vi "_calc_IFoutput.vi"(11 "Calc_IFout":T1={"Th"=299.0, "Tc"=83.0, "BW (MHz)"=40.0, "NS_output_data"=path "L:/cartridge/assembly/SN03/03-13/110628_WCADSB_P0/YIG_938.00_120_110628_WCADSB_P0aNS.csv", "Rx_output_data"=path "L:/cartridge/assembly/SN03/03-13/110628_WCADSB_P0/YIG_802.00_120_110628_WCADSB_P0m.csv", "NS_ENR"=path "Z:/Labview_ALMA/MIX10/110627_IFBOX/NS_ENR_44421726.csv", "SAVE"=TRUE, "IFB_NS_AMP(filename)"="", "IFB_INPUT_CBL(filename) "=""}) -> (1 "出力文字列":string, 3 "Calc_IFout 2":T1={"Th"=299.0, "Tc"=83.0, "BW (MHz)"=40.0, "NS_output_data"=path "L:/cartridge/assembly/SN03/03-13/110628_WCADSB_P0/YIG_938.00_120_110628_WCADSB_P0aNS.csv", "Rx_output_data"=path "L:/cartridge/assembly/SN03/03-13/110628_WCADSB_P0/YIG_802.00_120_110628_WCADSB_P0m.csv", "NS_ENR"=path "Z:/Labview_ALMA/MIX10/110627_IFBOX/NS_ENR_44421726.csv", "SAVE"=TRUE, "IFB_NS_AMP(filename)"="", "IFB_INPUT_CBL(filename) "=""})   [LabVIEW 2017]
uses:
  <vilib>/Utility/file.llb/Read From Spreadsheet File (DBL).vi
  <vilib>/Utility/file.llb/Read From Spreadsheet File (string).vi
  Instance           2 22Saved   _calc_IFoutput .vi
  Instance           3 22Saved   _calc_IFoutput .vi
  Instance           4 22Saved   _calc_IFoutput .vi
  Instance           5 22Saved   _calc_IFoutput .vi
  Instance           6 22Saved   _calc_IFoutput .vi
  <vilib>/express/express shared/transition.llb/Dynamic To Waveform Array.vi
  <vilib>/express/express arith-compare/Formula/Block/exnFormulaBlock how many pts in the wave.vi
  <vilib>/express/express shared/ex_Modify Signal Name.vi
  <vilib>/express/express shared/transition.llb/Waveform Array To Dynamic.vi
  Instance          14 22Saved   _calc_IFoutput .vi
  Instance          13 22Saved   _calc_IFoutput .vi
  Instance           8 22Saved   _calc_IFoutput .vi
  Instance          27 22Saved   _calc_IFoutput .vi
  Instance          25 22Saved   _calc_IFoutput .vi
  Instance          24 22Saved   _calc_IFoutput .vi
  Instance          23 22Saved   _calc_IFoutput .vi
  Instance           9 22Saved   _calc_IFoutput .vi
  <vilib>/express/express arith-compare/Formula/XNode/ExpressFormulaBlockNode.xnode
  <vilib>/gmath/NI_Gmath.lvlib
panel:
  out "配列 2":dbl[][](array[numeric])=[[3.8, -17.12272, -18.81083, -15.55195, -27.42913, -0.8529618823529413, 2646.4699989426, 27.159200000349998, 21.830696906606043], [3.85, -17.57263, -19.57423, -15.61331, -27.39271, -0.8547822352941177, 2630.0700003280003, 27.222799998728, 21.827656711269793], [3.9, -17.18393, -19.46044, -15.25915, -26.95194, -0.8662073529411765, 2669.6499992084, 27.104500002366002, 21.82485128829734], [3.95, -16.20817, -18.50417, -14.57025, -26.2268, -0.8667218823529415, 2730.9599987738, 27.08000000049, 21.822294447827726], [4.0, -15.03429, -17.26599, -13.90883, -25.64848, -0.882467, 2669.1500012362003, 27.084199999916, 21.82], [4.05, -14.82404, -17.0148, -13.89065, -25.63071, -0.881857, 2537.9100026248, 27.120499999274, 21.817975444814163], [4.1, -14.67198, -16.88321, -13.75199, -25.74328, -0.8925589411764706, 2521.6700003248, 26.984300002724, 21.81620304171403], [4.15, -13.82526, -16.05723, -13.35155, -25.22083, -0.8985360624999998, 2529.2999998474, 26.948000000726, 21.81465874000436], [4.2, -13.29308, -15.43659, -13.22012, -25.15282, -0.901060705882353, 2508.1700004226, 26.933300000294, 21.81331848898993], [4.25, -13.22027, -15.33436, -13.24037, -25.05297, -0.9175218823529412, 2527.4499996144, 26.893400000798, 21.812158237975495], [4.3, -13.31871, -15.44813, -13.02047, -24.85233, -0.9171115294117648, 2617.4499981999998, 26.800200001864, 21.81115393626583], [4.35, -13.69981, -15.96198, -12.64103, -24.38364, -0.9331128235294116, 2655.3199992426003, 26.946899997065998, 21.810281533165693], [4.4, -13.88617, -16.39624, -12.56773, -24.29817, -0.9225989999999998, 2612.6100008542003, 26.89840000097, 21.809516977979857], [4.45, -14.02675, -16.71935, -12.80309, -24.58885, -0.9326420000000001, 2578.7800006766, 26.85540000086, 21.808836220013085], [4.5, -14.20917, -16.89711, -12.97901, -24.88372, -0.9390088823529412, 2494.6900016818004, 26.752700002054002, 21.808215208570147], [4.55, -14.08214, -16.69081, -12.94844, -24.93315, -0.948472375, 2435.9600011746, 26.64920000207, 21.807629892955802], [4.6, -14.17748, -16.75517, -13.06879, -25.00575, -0.9494775294117647, 2433.2400000544, 26.427400004436, 21.80705622247482], [4.65, -14.20809, -16.81901, -13.13087, -25.16717, -0.9524575882352941, 2443.0399998039998, 26.363500001278, 21.80647014643197], [4.7, -13.73884, -16.38887, -13.13099, -25.03512, -0.9655740588235294, 2433.8500001838, 26.45199999823, 21.805847614132016], [4.75, -13.52419, -16.15298, -13.15192, -24.9704, -0.9653059411764703, 2516.0199983566, 26.454299999954, 21.805164574879722], [4.8, -13.5663, -16.20232, -13.10517, -24.80095, -0.976770176470588, 2562.8099990642, 26.343600002214, 21.804396977979856], [4.85, -13.97629, -16.65383, -13.30715, -25.25404, -0.9746549411764707, 2478.4000016882, 26.311400000644, 21.803520772737187], [4.9, -14.61364, -17.38417, -13.78671, -25.66877, -0.988881117647059, 2394.9800016684003, 26.140100003426, 21.802511908456477], [4.95, -14.4268, -17.25931, -13.81209, -25.80221, -0.9904888125, 2426.7199993652, 26.145399999894, 21.801346334442492], [5.0, -13.84685, -16.67325, -13.20797, -25.09457, -0.9986477647058825, 2402.3700004869997, 26.405599994796, 21.8], [5.05, -14.28601, -17.05717, -13.45101, -25.54052, -1.004, 2304.7500019524, 26.325300001606, 21.798457844989954], [5.1, -14.91876, -17.64101, -13.96415, -26.02207, -1.0068823529411761, 2324.9199995966, 26.481899996868, 21.796740771498058], [5.15, -15.14906, -17.85047, -14.16308, -26.17572, -1.0180588235294117, 2408.1599983352, 26.271100004216002, 21.794878672166195], [5.2, -14.66069, -17.39484, -13.82115, -25.80543, -1.0208823529411764, 2393.2200002987997, 26.329699998827998, 21.792901439636257], [5.25, -13.73691, -16.45963, -13.31747, -25.36704, -1.028, 2326.370001337, 26.25120000157, 21.790838966550133], [5.3, -13.70664, -16.41934, -13.34713, -25.41262, -1.0291176470588232, 2366.9299991887997, 26.28519999932, 21.78872114554971], [5.35, -14.26567, -16.97919, -13.7311, -25.69348, -1.042, 2383.6799996649997, 26.357999998544, 21.78657786927688], [5.4, -14.42577, -17.17993, -13.89956, -26.00954, -1.046, 2311.580001442, 26.332800000503997, 21.784439030373523], [5.45, -14.3035, -17.10186, -13.87839, -26.01249, -1.0538235294117648, 2274.08000075, 26.241800001820003, 21.782334521481534], [5.5, -14.13436, -16.92141, -13.94402, -26.09274, -1.0542500000000001, 2305.5199993712, 26.224000000356, 21.780294235242803], [5.55, -14.09064, -16.88934, -13.93655, -25.97309, -1.0640588235294117, 2314.2099998262, 26.143600001608, 21.778348064299216], [5.6, -14.13487, -16.88146, -13.83602, -26.02727, -1.0725882352941176, 2258.5000011142, 26.194499998982, 21.776525901292658], [5.65, -14.0179, -16.75543, -13.67357, -25.85477, -1.0641764705882353, 2249.6300001774002, 26.303699997816, 21.774857638865026], [5.7, -13.742, -16.4761, -13.49645, -25.65245, -1.085294117647059, 2312.4099987443997, 26.495899996156, 21.7733731696582], [5.75, -13.63401, -16.37811, -13.62051, -25.66763, -1.0879411764705882, 2296.9000003102, 26.546799998982, 21.77210238631407], [5.8, -13.9966, -16.7347, -14.08119, -26.28417, -1.0975294117647059, 2229.90000134, 26.494200001052, 21.77107518147453], [5.85, -14.3776, -17.12208, -14.29554, -26.5205, -1.0957647058823532, 2219.9900001981996, 26.459700000690002, 21.770321447781463], [5.9, -14.33998, -17.0836, -14.21864, -26.41191, -1.0961250000000002, 2230.8999997818, 26.353800002118, 21.76987107787676], [5.95, -14.05573, -16.80771, -13.83659, -26.01129, -1.106764705882353, 2262.3899993702, 26.544199996192, 21.76975396440231], [6.0, -14.15222, -16.88773, -14.02318, -26.27665, -1.110529411764706, 2218.8600008706003, 26.523000000424, 21.77], [6.05, -14.42877, -17.16834, -14.46916, -26.71696, -1.1207647058823527, 2201.7700003418, 26.482100000818, 21.770629425226016], [6.1, -14.82458, -17.54857, -14.74361, -26.94142, -1.1145882352941179, 2213.8099997592, 26.528199999077998, 21.77162387229374], [6.15, -14.43141, -17.15023, -14.50576, -26.74506, -1.1284117647058822, 2219.209999892, 26.454400001476, 21.77295532133086], [6.2, -13.88065, -16.61938, -14.37111, -26.68039, -1.128235294117647, 2179.0500008032004, 26.372000001648, 21.77459575246504], [6.25, -13.64365, -16.3979, -14.22502, -26.5427, -1.135764705882353, 2168.7100002068, 26.34000000064, 21.77651714582397], [6.3, -13.8741, -16.64741, -14.49609, -26.71762, -1.14025, 2200.3899993664, 26.582799995143997, 21.77869148153533], [6.35, -14.26957, -17.0322, -14.86186, -27.19956, -1.1440588235294114, 2204.6199999154, 26.591799999819997, 21.781090739726796], [6.4, -15.05829, -17.80809, -15.42064, -27.71206, -1.1539411764705882, 2184.0000004124, 26.470100002434, 21.78368690052605], [6.45, -14.96881, -17.71266, -15.38201, -27.65482, -1.1564705882352941, 2195.249999775, 26.481999999762, 21.786451944060772], [6.5, -14.62204, -17.38934, -15.02896, -27.20097, -1.1578823529411766, 2242.3699990575997, 26.306800003503998, 21.789357850458643], [6.55, -14.93231, -17.69407, -15.10335, -27.40647, -1.164235294117647, 2205.1300007448003, 26.310299999930002, 21.79237659984734], [6.6, -15.6833, -18.43714, -15.87043, -28.20904, -1.172, 2152.5300010520004, 26.339899999408, 21.795480172354544], [6.65, -16.11679, -18.87216, -16.20987, -28.58401, -1.1799411764705883, 2167.9899996908, 26.356799999661998, 21.798640548107933], [6.7, -15.71971, -18.45462, -15.76916, -28.0619, -1.185, 2201.939999321, 26.396499999206, 21.80182970723519], [6.75, -15.0464, -17.78941, -15.52487, -27.82688, -1.195, 2182.7000003847998, 26.399599999938, 21.805019629863992], [6.8, -15.48116, -18.24106, -16.05464, -28.38039, -1.2004117647058823, 2165.3400003472, 26.28360000232, 21.808182296122023], [6.85, -16.22272, -18.99162, -16.63654, -28.97924, -1.201, 2225.439998798, 26.274900000174, 21.81128968613696], [6.9, -15.67766, -18.42345, -16.38983, -28.69264, -1.2098823529411764, 2234.0299998282003, 26.270200000094, 21.814313780036482], [6.95, -15.36656, -18.07411, -15.9862, -28.27599, -1.2114117647058824, 2165.6200013682, 26.381899997766002, 21.817226557948267], [7.0, -15.74528, -18.46492, -16.29495, -28.63586, -1.218, 2163.1900000486003, 26.272700002184, 21.82], [7.05, -16.00173, -18.75385, -16.78861, -29.11719, -1.2230588235294118, 2187.8999995058, 26.169500002063998, 21.82260695410598], [7.1, -15.95475, -18.70909, -16.46813, -28.80718, -1.2295882352941179, 2186.0500000370002, 26.233599998718, 21.825023739326973], [7.15, -15.74736, -18.51188, -16.0888, -28.41011, -1.228, 2172.6600002677997, 26.140200001868, 21.827227542510375], [7.2, -15.79896, -18.55205, -16.49574, -28.80938, -1.2389411764705882, 2190.1299996506, 26.035800002088, 21.82919555050358], [7.25, -16.55221, -19.29029, -17.09613, -29.38037, -1.2441250000000001, 2230.579999191, 25.944300001829998, 21.830904950153982], [7.3, -16.63515, -19.36656, -17.1755, -29.45088, -1.2501764705882352, 2201.3800005840003, 26.127399996338003, 21.83233292830897], [7.35, -16.28817, -19.02285, -17.12399, -29.45578, -1.2507058823529413, 2186.5600002964, 26.014300002261997, 21.833456671815934], [7.4, -15.91257, -18.66145, -16.74209, -29.02037, -1.2591176470588235, 2205.0399996304, 26.029399999698, 21.834253367522273], [7.45, -15.41844, -18.14403, -16.48895, -28.79334, -1.2650588235294118, 2206.9099999626, 25.964200001304, 21.83470020227537], [7.5, -15.41264, -18.10839, -16.57757, -28.91563, -1.273764705882353, 2195.2200002338, 26.019099998902, 21.834774362922627], [7.55, -15.98175, -18.66501, -16.9447, -29.22746, -1.2748235294117647, 2200.019999904, 25.824000003902, 21.834453036311427], [7.6, -15.94066, -18.66749, -17.16323, -29.42903, -1.2809411764705882, 2244.7899991045997, 25.813600000208, 21.833713409289167], [7.65, -15.86338, -18.63036, -17.30867, -29.55716, -1.2772500000000002, 2247.2699999504, 25.856499999142, 21.83253266870324], [7.7, -15.93995, -18.73317, -17.33017, -29.58961, -1.2859411764705884, 2238.1100001832, 25.730900002511998, 21.83088800140104], [7.75, -15.60121, -18.40257, -17.32444, -29.63481, -1.299588235294118, 2218.8700003848, 25.69040000081, 21.828756594229954], [7.8, -15.52939, -18.3085, -17.34604, -29.61109, -1.2968235294117643, 2243.669999504, 25.680500000198, 21.82611563403738], [7.85, -15.91931, -18.69063, -17.7087, -29.96924, -1.3002352941176467, 2245.9399999546, 25.647100000667997, 21.8229423076707], [7.9, -16.06734, -18.84154, -18.21152, -30.51118, -1.3056250000000003, 2218.990000539, 25.507500002792, 21.819213801977316], [7.95, -16.2394, -19.01631, -18.39538, -30.77489, -1.313764705882353, 2222.539999929, 25.53849999938, 21.81490730380462], [8.0, -16.0832, -18.82693, -18.18621, -30.42877, -1.3231176470588235, 2253.7699993754, 25.421100002348, 21.81], [8.05, -15.9397, -18.65948, -18.21682, -30.46989, -1.332941176470588, 2276.81, 25.2307, 21.804486508350074], [8.1, -16.44804, -19.16853, -18.58308, -30.82861, -1.335, 2261.15, 25.2839, 21.79843117039837], [8.15, -16.97081, -19.72537, -19.0693, -31.4089, -1.3383529411764703, 2262.78, 25.2973, 21.79191575862764], [8.2, -16.87192, -19.67071, -19.41342, -31.67662, -1.348647058823529, 2301.63, 25.0593, 21.78502204552063], [8.25, -17.21139, -20.03537, -19.67853, -31.95149, -1.3514117647058825, 2289.19, 24.9943, 21.777831803560098], [8.3, -17.29203, -20.11014, -19.70503, -32.02495, -1.352470588235294, 2259.82, 25.224, 21.77042680522879], [8.35, -16.73358, -19.52565, -19.51154, -31.79005, -1.357705882352941, 2266.94, 24.9458, 21.76288882300946], [8.4, -16.47973, -19.26356, -19.55496, -31.8567, -1.365235294117647, 2296.06, 24.8175, 21.75529962938486], [8.45, -16.96765, -19.74245, -20.13428, -32.43519, -1.3692499999999999, 2317.78, 24.8136, 21.747740996837745], [8.5, -17.89289, -20.67773, -21.16278, -33.47596, -1.377, 2296.65, 24.8236, 21.740294697850857], [8.55, -18.31942, -21.11132, -21.53435, -33.99178, -1.377882352941177, 2303.42, 24.7167, 21.73304250490695], [8.6, -17.91342, -20.68657, -21.06001, -33.3284, -1.3864117647058825, 2312.28, 24.5475, 21.72606619048878], [8.65, -17.50286, -20.31712, -20.86753, -33.1991, -1.3915882352941176, 2326.39, 24.57, 21.719447527079094], [8.7, -17.7744, -20.60603, -21.46811, -33.89479, -1.3978823529411766, 2298.81, 24.1647, 21.713268287160645], [8.75, -17.86462, -20.69869, -21.66053, -34.15056, -1.4036470588235284, 2302.5, 24.3807, 21.707610243216184], [8.8, -17.71743, -20.57318, -21.35601, -33.74465, -1.4073529411764707, 2313.14, 24.5441, 21.702555167728462], [8.85, -17.94226, -20.78062, -21.59592, -34.02443, -1.4161875, 2345.93, 24.4626, 21.698184833180232], [8.9, -18.34472, -21.16955, -22.16719, -34.56456, -1.4160588235294116, 2339.53, 24.3008, 21.694581012054247], [8.95, -18.04812, -20.86419, -21.99622, -34.46492, -1.4309411764705886, 2338.73, 24.441, 21.69182547683325], [9.0, -17.40652, -20.21983, -21.48231, -33.78672, -1.4215882352941176, 2358.4, 24.3139, 21.69], [9.05, -17.24231, -20.07737, -21.48494, -33.82899, -1.4349411764705877, 2366.74, 24.1072, 21.689155762493723], [9.1, -17.74864, -20.56868, -21.94918, -34.39316, -1.4335882352941178, 2338.76, 24.3848, 21.689221579079543], [9.15, -18.4194, -21.25906, -22.30343, -34.74111, -1.453, 2315.94, 24.6737, 21.690095672979066], [9.2, -18.22584, -21.06735, -22.19776, -34.35875, -1.451705882352941, 2343.85, 24.5305, 21.69167626741389], [9.25, -17.60283, -20.47247, -21.72121, -33.8754, -1.4561250000000001, 2374.94, 24.293, 21.69386158560562], [9.3, -17.285, -20.1526, -21.26908, -33.42764, -1.4694117647058822, 2365.34, 24.4681, 21.69654985077586], [9.35, -17.46603, -20.32564, -21.38399, -33.71154, -1.4681764705882352, 2354.91, 24.3401, 21.699639286146212], [9.4, -17.69275, -20.52774, -21.7712, -34.03559, -1.4925882352941173, 2368.34, 24.4059, 21.703028114938277], [9.45, -17.89483, -20.70066, -21.80327, -33.93689, -1.473, 2362.78, 24.6405, 21.706614560373655], [9.5, -17.75022, -20.53087, -21.69907, -34.00557, -1.507411764705883, 2338.42, 24.6167, 21.710296845673955], [9.55, -17.66432, -20.45212, -21.90227, -34.10663, -1.4951764705882342, 2333.22, 24.5527, 21.713973194060774], [9.6, -17.65736, -20.44671, -21.78109, -33.9852, -1.522470588235294, 2332.23, 24.4424, 21.717541828755717], [9.65, -17.73314, -20.5128, -21.7289, -33.99685, -1.517823529411764, 2328.62, 24.6084, 21.720900972980388], [9.7, -17.4669, -20.25952, -21.67133, -33.91276, -1.525588235294116, 2351.26, 24.2804, 21.723948849956383], [9.75, -17.76851, -20.58019, -22.0069, -34.18419, -1.5647058823529412, 2359.86, 24.4864, 21.72658368290531], [9.8, -18.45745, -21.3164, -22.66344, -34.81685, -1.5282499999999999, 2394.51, 24.4116, 21.72870369504877], [9.85, -18.74849, -21.60512, -23.1135, -35.51059, -1.5908235294117645, 2378.32, 24.3508, 21.73020710960837], [9.9, -18.03912, -20.85912, -22.19721, -34.52363, -1.5453529411764708, 2394.59, 24.2431, 21.730992149805704], [9.95, -17.9064, -20.68631, -21.64287, -33.76706, -1.6109999999999993, 2382.76, 24.4119, 21.730957038862382], [10.0, -18.76585, -21.52492, -22.34931, -34.56586, -1.5900588235294104, 2349.48, 24.4835, 21.73], [10.05, -19.5962, -22.32853, -22.9941, -35.31366, -1.6072352941176506, 2367.23, 24.3783, 21.72805419167504], [10.1, -19.6706, -22.4559, -22.82671, -35.05968, -1.6390588235294121, 2371.78, 24.5145, 21.72519251328346], [10.15, -19.60253, -22.38713, -22.75759, -35.06578, -1.594882352941177, 2400.96, 24.3435, 21.721522799456107], [10.2, -19.78752, -22.57098, -23.06087, -35.44369, -1.681875, 2420.45, 24.0411, 21.71715288482381], [10.25, -20.0526, -22.84692, -23.63574, -35.82155, -1.6011764705882354, 2439.32, 23.8385, 21.712190604017422], [10.3, -19.54974, -22.37162, -23.29077, -35.54749, -1.6889411764705888, 2425.46, 24.0043, 21.70674379166777], [10.35, -19.60772, -22.45374, -23.18082, -35.44497, -1.6339411764705871, 2402.21, 24.136, 21.700920282405693], [10.4, -19.77289, -22.58667, -23.44011, -35.6872, -1.6639411764705916, 2403.53, 24.1481, 21.69482791086204], [10.45, -19.79049, -22.58858, -23.37076, -35.6931, -1.6936470588235286, 2410.86, 24.2845, 21.688574511667635], [10.5, -19.04526, -21.81113, -22.73856, -34.75031, -1.6280000000000006, 2432.24, 24.1535, 21.68226791945333], [10.55, -18.56993, -21.3308, -22.71269, -34.42597, -1.7282941176470574, 2457.87, 23.9651, 21.676015968849956], [10.6, -18.81393, -21.59022, -23.3418, -35.09374, -1.627000000000001, 2472.89, 23.7868, 21.669926494488355], [10.65, -19.22983, -22.00177, -23.51241, -35.50699, -1.7109411764705882, 2463.24, 23.8037, 21.664107330999364], [10.7, -19.31875, -22.05797, -23.32962, -35.59218, -1.6540588235294145, 2430.32, 23.8234, 21.658666313013825], [10.75, -19.05511, -21.80451, -23.11849, -35.37068, -1.6625882352941161, 2456.31, 23.8229, 21.653711275162575], [10.8, -19.3566, -22.10467, -23.36395, -35.42174, -1.644, 2526.85, 23.8448, 21.64935005207645], [10.85, -19.0206, -21.80983, -23.26736, -35.08837, -1.653941176470586, 2539.44, 23.6902, 21.645690478386292], [10.9, -18.31242, -21.08287, -22.35121, -34.319, -1.678058823529411, 2516.98, 23.7731, 21.642840388722938], [10.95, -18.58308, -21.32811, -22.20398, -34.26554, -1.6376470588235292, 2511.94, 23.7372, 21.64090761771723], [11.0, -19.33065, -22.06466, -22.81771, -34.93946, -1.6834705882352938, 2495.74, 23.8567, 21.64], [11.05, -19.70611, -22.43568, -23.07443, -35.23765, -1.6487058823529408, 2471.76, 23.7069, 21.64017747080613], [11.1, -19.03199, -21.75445, -22.37182, -34.36297, -1.6840588235294118, 2484.68, 23.978, 21.64130836778662], [11.15, -18.20851, -20.94228, -21.81273, -33.92755, -1.65975, 2530.13, 23.6561, 21.643213129196518], [11.2, -18.60047, -21.36138, -22.13935, -34.33841, -1.7035294117647042, 2549.97, 23.6568, 21.645712193290862], [11.25, -19.51813, -22.27067, -22.85502, -34.9773, -1.6814705882352947, 2588.62, 23.5463, 21.6486259983247], [11.3, -20.00388, -22.73884, -23.1136, -35.31568, -1.7118823529411817, 2547.84, 23.759, 21.651774982553068], [11.35, -20.09303, -22.81332, -23.00719, -35.05995, -1.7251176470588228, 2534.41, 23.8176, 21.654979584231015], [11.4, -19.73824, -22.45692, -22.58862, -34.67323, -1.7182352941176506, 2543.99, 23.8915, 21.658060241613576], [11.45, -19.50205, -22.22064, -22.28212, -34.3972, -1.75829411764706, 2558.35, 23.9421, 21.660837392955802], [11.5, -19.44096, -22.15222, -22.1292, -34.22024, -1.7096470588235253, 2566.32, 23.8669, 21.663131476512728], [11.55, -19.53986, -22.21978, -22.16747, -34.08258, -1.805937499999999, 2585.21, 23.691, 21.664762930539403], [11.6, -19.66825, -22.31744, -22.50284, -34.28826, -1.7306470588235299, 2620.79, 23.6435, 21.665552193290864], [11.65, -20.25282, -22.89179, -22.68607, -34.6127, -1.833705882352942, 2632.79, 23.8005, 21.665319703022153], [11.7, -20.71909, -23.33487, -22.77796, -34.75574, -1.7838235294117686, 2608.38, 23.9055, 21.663885897988315], [11.75, -20.60419, -23.22526, -22.42747, -34.3851, -1.7971764705882394, 2594.61, 24.0102, 21.661071216444395], [11.8, -19.96298, -22.55664, -21.58718, -33.45363, -1.8430588235294112, 2639.94, 23.9067, 21.656696096645433], [11.85, -19.76787, -22.40006, -21.42269, -33.29006, -1.7760588235294126, 2643.51, 23.9414, 21.650580976846467], [11.9, -20.8505, -23.49592, -22.22725, -34.22635, -1.8767647058823524, 2626.67, 23.9677, 21.642546295302548], [11.95, -21.60192, -24.17152, -22.54207, -34.5773, -1.7737499999999975, 2639.97, 23.9508, 21.63241249026871], [12.0, -21.64507, -24.22899, -22.299, -34.30385, -1.8910588235294117, 2735.39, 23.7742, 21.62], [12.05, -21.23121, -23.79945, -21.79121, -33.84, -1.7987058823529407, 2735.72, 24.015, 21.60517967510045], [12.1, -20.95311, -23.50938, -21.58213, -33.39882, -1.879823529411763, 2675.38, 24.0166, 21.588024015570067], [12.15, -20.98547, -23.59292, -21.93953, -33.86782, -1.885, 2668.38, 24.2213, 21.56865593375783], [12.2, -20.95372, -23.58369, -22.31312, -34.16981, -1.8179411764705862, 2763.59, 23.8837, 21.54719834201274]]
  in  "タブ制御器":enum32{"YIGファイル", "配列"}(tab)
  out "Trx(K)":dbl=258.9214466673217 format="%#_5g"
  out "PrxCold(dBm)":dbl=-6.962263655715082 format="%#_4g"
  out "PrxHOT(dBm)":dbl=-4.835796517513394 format="%#_4g"
  out "XYグラフ 4":cluster{"データ配列":dbl[], "データ配列":dbl[]}[](graph)=[{"データ配列"=[4.0, 4.1, 4.2, 4.3, 4.4, 4.5, 4.6, 4.7, 4.8, 4.9, 5.0, 5.1, 5.2, 5.3, 5.4, 5.5, 5.6, 5.7, 5.8, 5.9, 6.0, 6.1, 6.2, 6.3, 6.4, 6.5, 6.6, 6.7, 6.8, 6.9, 7.0, 7.1, 7.2, 7.3, 7.4, 7.5, 7.6, 7.7, 7.8, 7.9, 8.0, 8.1, 8.2, 8.3, 8.4, 8.5, 8.6, 8.7, 8.8, 8.9, 9.0, 9.1, 9.2, 9.3, 9.4, 9.5, 9.6, 9.7, 9.8, 9.9, 10.0, 10.1, 10.2, 10.3, 10.4, 10.5, 10.6, 10.7, 10.8, 10.9, 11.0, 11.1, 11.2, 11.3, 11.4, 11.5, 11.6, 11.7, 11.8, 11.9, 12.0], "データ配列"=[-42.304058133402506, -42.04170104561826, -42.25769085666673, -42.31033056902308, -42.699370793354305, -42.9673333159231, -42.837630586787604, -42.94984868225228, -43.07707400925531, -42.66207963493079, -42.98011802522254, -43.45648977225463, -43.280806658564245, -43.634589212892486, -44.018645325326226, -43.81372941546897, -43.76980228766497, -43.96918926175765, -43.986226970817, -44.024745724653854, -44.2990635530348, -44.094645933336906, -43.98832153150062, -43.946678895226086, -43.67736451771449, -43.85248156438922, -44.072831890236266, -44.26537276912129, -44.13913616205879, -44.009433614744594, -43.918231331259655, -44.030884167315875, -44.31466142206972, -44.493289418320245, -44.49089464719869, -44.7392295395062, -44.42057403155067, -44.2279010527397, -44.53456965048816, -44.33192110058992, -44.35971000898137, -44.75547143915319, -44.79102247770662, -44.468178244294656, -44.43278840023204, -44.46644883392027, -44.11964718633102, -44.16930583654094, -44.32129391903585, -44.37722482951502, -44.03954965889642, -43.91817166456329, -44.19873556734652, -43.99862590961723, -43.84111258473843, -44.21531647455938, -44.297269712777904, -43.75561086527098, -43.918462838542595, -43.99076991963976, -43.63530516028899, -43.90978604302725, -43.952711025560276, -43.90897239791697, -44.08618137809738, -43.893909627344996, -44.15642536559794, -44.10336227759402, -44.06279401495067, -44.20067317922716, -44.219315282199645, -44.486166112971304, -44.20807200459492, -43.97480625686816, -44.12732399906333, -44.380180854477324, -44.765220199391514, -45.03550740084957, -45.01000250395328, -45.301369374868585, -44.81874285356317]}, {"データ配列"=[4.0, 4.1, 4.2, 4.3, 4.4, 4.5, 4.6, 4.7, 4.8, 4.9, 5.0, 5.1, 5.2, 5.3, 5.4, 5.5, 5.6, 5.7, 5.8, 5.9, 6.0, 6.1, 6.2, 6.3, 6.4, 6.5, 6.6, 6.7, 6.8, 6.9, 7.0, 7.1, 7.2, 7.3, 7.4, 7.5, 7.6, 7.7, 7.8, 7.9, 8.0, 8.1, 8.2, 8.3, 8.4, 8.5, 8.6, 8.7, 8.8, 8.9, 9.0, 9.1, 9.2, 9.3, 9.4, 9.5, 9.6, 9.7, 9.8, 9.9, 10.0, 10.1, 10.2, 10.3, 10.4, 10.5, 10.6, 10.7, 10.8, 10.9, 11.0, 11.1, 11.2, 11.3, 11.4, 11.5, 11.6, 11.7, 11.8, 11.9, 12.0], "データ配列"=[-43.9040581334025, -43.66170104561826, -43.947690856666725, -43.87033056902308, -44.379370793354305, -44.757333315923105, -44.477630586787605, -44.58984868225228, -44.78707400925531, -44.21207963493079, -44.68011802522254, -45.33648977225463, -45.060806658564246, -45.55458921289249, -46.18864532532622, -45.98372941546897, -46.049802287664974, -46.34918926175765, -46.16622697081701, -46.15474572465385, -46.6590635530348, -46.49464593333691, -46.43832153150062, -46.34667889522608, -45.937364517714485, -46.14248156438922, -46.48283189023627, -46.65537276912129, -46.519136162058786, -46.3194336147446, -46.168231331259655, -46.420884167315876, -46.80466142206972, -46.87328941832025, -46.65089464719868, -46.999229539506196, -46.72057403155067, -46.4779010527397, -46.89456965048816, -46.55192110058992, -46.40971000898137, -46.96547143915319, -47.021022477706616, -46.65817824429465, -46.64278840023205, -46.55644883392027, -46.19964718633102, -46.32930583654094, -46.481293919035856, -46.537224829515026, -46.10954965889642, -45.968171664563286, -46.408735567346525, -46.24862590961723, -46.01111258473843, -46.43531647455938, -46.5072697127779, -45.89561086527098, -46.2284628385426, -46.34076991963976, -45.88530516028899, -46.20978604302725, -46.32271102556028, -46.32897239791697, -46.516181378097386, -46.353909627345, -46.56642536559794, -46.523362277594025, -46.51279401495067, -46.540673179227156, -46.55931528219965, -46.8361661129713, -46.45807200459492, -46.24480625686816, -46.347323999063335, -46.52018085447732, -46.865220199391516, -47.12550740084957, -47.14000250395328, -47.42136937486859, -46.89874285356318]}, {"データ配列"=[4.0, 4.1, 4.2, 4.3, 4.4, 4.5, 4.6, 4.7, 4.8, 4.9, 5.0, 5.1, 5.2, 5.3, 5.4, 5.5, 5.6, 5.7, 5.8, 5.9, 6.0, 6.1, 6.2, 6.3, 6.4, 6.5, 6.6, 6.7, 6.8, 6.9, 7.0, 7.1, 7.2, 7.3, 7.4, 7.5, 7.6, 7.7, 7.8, 7.9, 8.0, 8.1, 8.2, 8.3, 8.4, 8.5, 8.6, 8.7, 8.8, 8.9, 9.0, 9.1, 9.2, 9.3, 9.4, 9.5, 9.6, 9.7, 9.8, 9.9, 10.0, 10.1, 10.2, 10.3, 10.4, 10.5, 10.6, 10.7, 10.8, 10.9, 11.0, 11.1, 11.2, 11.3, 11.4, 11.5, 11.6, 11.7, 11.8, 11.9, 12.0], "データ配列"=[401.9140426735799, 394.75812785452376, 371.0614536288631, 416.7826185394593, 374.3243326980722, 340.4628582128464, 387.77874142440936, 387.77874142440936, 364.6516148294494, 420.62099002242826, 367.83744166083335, 315.7443592189742, 343.3659439767455, 305.51322405740643, 250.24981952690112, 250.24981952690044, 229.84356141214752, 212.96486468500444, 248.30775543404707, 258.20422615941976, 216.22344244475124, 209.76193734579428, 201.9891414146812, 209.76193734579485, 233.40282283656907, 228.08777292672426, 208.1809094089769, 211.35653207271164, 212.96486468500444, 224.62284785774372, 235.20671980907528, 211.35653207271164, 196.001465831908, 212.96486468500444, 252.21024001848184, 233.40282283656907, 226.34760271499096, 235.20671980907528, 216.22344244475124, 240.71810018385082, 275.0632414827429, 242.5892088875253, 238.86413487820636, 246.3837961976696, 242.5892088875253, 266.4693030754984, 268.58621557379115, 252.21024001848184, 252.21024001848184, 252.21024001848184, 270.7239727210061, 275.0632414827429, 242.5892088875253, 235.20671980907528, 250.24981952690112, 240.71810018385082, 242.58920888752598, 256.18717987357735, 224.62284785774372, 217.8740444657678, 235.20671980907528, 226.34760271499096, 214.5871091652999, 206.61327999467903, 205.05888360483368, 200.47347796194887, 208.1809094089769, 206.6132799946785, 201.98914141468066, 219.5390982463626, 219.5390982463626, 217.8740444657678, 235.20671980907528, 231.61517466578167, 240.71810018385014, 256.18717987357803, 264.3729373605166, 266.4693030754984, 258.2042261594205, 260.2406829166549, 268.5862155737904]}]
  out "XYグラフ 7":cluster{"データ配列":dbl[], "データ配列":dbl[]}[](graph)=[{"データ配列"=[4.0, 4.1, 4.2, 4.3, 4.4, 4.5, 4.6, 4.7, 4.8, 4.9, 5.0, 5.1, 5.2, 5.3, 5.4, 5.5, 5.6, 5.7, 5.8, 5.9, 6.0, 6.1, 6.2, 6.3, 6.4, 6.5, 6.6, 6.7, 6.8, 6.9, 7.0, 7.1, 7.2, 7.3, 7.4, 7.5, 7.6, 7.7, 7.8, 7.9, 8.0, 8.1, 8.2, 8.3, 8.4, 8.5, 8.6, 8.7, 8.8, 8.9, 9.0, 9.1, 9.2, 9.3, 9.4, 9.5, 9.6, 9.7, 9.8, 9.9, 10.0, 10.1, 10.2, 10.3, 10.4, 10.5, 10.6, 10.7, 10.8, 10.9, 11.0, 11.1, 11.2, 11.3, 11.4, 11.5, 11.6, 11.7, 11.8, 11.9, 12.0], "データ配列"=[-42.304058133402506, -42.04170104561826, -42.25769085666673, -42.31033056902308, -42.699370793354305, -42.9673333159231, -42.837630586787604, -42.94984868225228, -43.07707400925531, -42.66207963493079, -42.98011802522254, -43.45648977225463, -43.280806658564245, -43.634589212892486, -44.018645325326226, -43.81372941546897, -43.76980228766497, -43.96918926175765, -43.986226970817, -44.024745724653854, -44.2990635530348, -44.094645933336906, -43.98832153150062, -43.946678895226086, -43.67736451771449, -43.85248156438922, -44.072831890236266, -44.26537276912129, -44.13913616205879, -44.009433614744594, -43.918231331259655, -44.030884167315875, -44.31466142206972, -44.493289418320245, -44.49089464719869, -44.7392295395062, -44.42057403155067, -44.2279010527397, -44.53456965048816, -44.33192110058992, -44.35971000898137, -44.75547143915319, -44.79102247770662, -44.468178244294656, -44.43278840023204, -44.46644883392027, -44.11964718633102, -44.16930583654094, -44.32129391903585, -44.37722482951502, -44.03954965889642, -43.91817166456329, -44.19873556734652, -43.99862590961723, -43.84111258473843, -44.21531647455938, -44.297269712777904, -43.75561086527098, -43.918462838542595, -43.99076991963976, -43.63530516028899, -43.90978604302725, -43.952711025560276, -43.90897239791697, -44.08618137809738, -43.893909627344996, -44.15642536559794, -44.10336227759402, -44.06279401495067, -44.20067317922716, -44.219315282199645, -44.486166112971304, -44.20807200459492, -43.97480625686816, -44.12732399906333, -44.380180854477324, -44.765220199391514, -45.03550740084957, -45.01000250395328, -45.301369374868585, -44.81874285356317]}, {"データ配列"=[4.0, 4.1, 4.2, 4.3, 4.4, 4.5, 4.6, 4.7, 4.8, 4.9, 5.0, 5.1, 5.2, 5.3, 5.4, 5.5, 5.6, 5.7, 5.8, 5.9, 6.0, 6.1, 6.2, 6.3, 6.4, 6.5, 6.6, 6.7, 6.8, 6.9, 7.0, 7.1, 7.2, 7.3, 7.4, 7.5, 7.6, 7.7, 7.8, 7.9, 8.0, 8.1, 8.2, 8.3, 8.4, 8.5, 8.6, 8.7, 8.8, 8.9, 9.0, 9.1, 9.2, 9.3, 9.4, 9.5, 9.6, 9.7, 9.8, 9.9, 10.0, 10.1, 10.2, 10.3, 10.4, 10.5, 10.6, 10.7, 10.8, 10.9, 11.0, 11.1, 11.2, 11.3, 11.4, 11.5, 11.6, 11.7, 11.8, 11.9, 12.0], "データ配列"=[0.0, 0.0, 0.0, 0.0, 0.0, 0.0, 0.0, 0.0, 0.0, 0.0, 1.9830446790355936, 2.2573625074165378, 2.0413726963680716, 1.988732984011719, 1.6369839181040078, 1.6369839181040078, 1.6369839181040078, 1.6369839181040078, 1.6369839181040078, 1.6369839181040078, 1.3189455278122608, 1.0182568944705537, 1.0182568944705537, 0.6800722091772329, 0.8159249006057578, 0.8159249006057578, 1.0618650217917107, 1.0618650217917107, 1.0618650217917107, 1.0618650217917107, 1.0618650217917107, 1.0618650217917107, 1.0781069214387031, 1.113657959992132, 1.113657959992132, 0.9385409133173965, 0.8727911464469642, 0.8727911464469642, 0.8727911464469642, 0.8727911464469642, 0.8727911464469642, 0.7601383103907438, 0.8728508131433301, 0.8728508131433301, 0.8728508131433301, 0.9499098929681864, 0.9499098929681864, 0.9499098929681864, 1.035411612435638, 1.035411612435638, 1.035411612435638, 1.1557173174176256, 1.1557173174176256, 0.8328730840056622, 0.8311436736312743, 0.8311436736312743, 0.7419196692260286, 0.7419196692260286, 0.7419196692260286, 0.7419196692260286, 0.6619645524889108, 0.6619645524889108, 0.8508609526823108, 0.8508609526823108, 0.8508609526823108, 0.8508609526823108, 0.8508609526823108, 1.1299150391025208, 1.4002022405605743, 1.4002022405605743, 1.6660642145795919, 0.0, 0.0, 0.0, 0.0, 0.0, 0.0, 0.0, 0.0, 0.0, 0.0]}]
  out "Inband PP":dbl=3.2596683292503243 format="%#_4g"
  out "文字列配列":string[][](array[string])=[[" 2011-06-28  15:04:04", " 2011-06-28  15:04:07", " 2011-06-28  15:04:09", " 2011-06-28  15:04:12", " 2011-06-28  15:04:15", " 2011-06-28  15:04:18", " 2011-06-28  15:04:21", " 2011-06-28  15:04:24", " 2011-06-28  15:04:27", " 2011-06-28  15:04:29", " 2011-06-28  15:04:32", " 2011-06-28  15:04:35", " 2011-06-28  15:04:38", " 2011-06-28  15:04:41", " 2011-06-28  15:04:44", " 2011-06-28  15:04:47", " 2011-06-28  15:04:50", " 2011-06-28  15:04:52", " 2011-06-28  15:04:55", " 2011-06-28  15:04:58", " 2011-06-28  15:05:01", " 2011-06-28  15:05:04", " 2011-06-28  15:05:07", " 2011-06-28  15:05:10", " 2011-06-28  15:05:12", " 2011-06-28  15:05:15", " 2011-06-28  15:05:18", " 2011-06-28  15:05:21", " 2011-06-28  15:05:24", " 2011-06-28  15:05:27", " 2011-06-28  15:05:30", " 2011-06-28  15:05:32", " 2011-06-28  15:05:35", " 2011-06-28  15:05:38", " 2011-06-28  15:05:41", " 2011-06-28  15:05:44", " 2011-06-28  15:05:47", " 2011-06-28  15:05:50", " 2011-06-28  15:05:52", " 2011-06-28  15:05:55", " 2011-06-28  15:05:58", " 2011-06-28  15:06:01", " 2011-06-28  15:06:04", " 2011-06-28  15:06:07", " 2011-06-28  15:06:10", " 2011-06-28  15:06:13", " 2011-06-28  15:06:15", " 2011-06-28  15:06:18", " 2011-06-28  15:06:21", " 2011-06-28  15:06:24", " 2011-06-28  15:06:27", " 2011-06-28  15:06:30", " 2011-06-28  15:06:33", " 2011-06-28  15:06:36", " 2011-06-28  15:06:38", " 2011-06-28  15:06:41", " 2011-06-28  15:06:44", " 2011-06-28  15:06:47", " 2011-06-28  15:06:50", " 2011-06-28  15:06:53", " 2011-06-28  15:06:56", " 2011-06-28  15:06:58", " 2011-06-28  15:07:01", " 2011-06-28  15:07:04", " 2011-06-28  15:07:07", " 2011-06-28  15:07:10", " 2011-06-28  15:07:13", " 2011-06-28  15:07:16", " 2011-06-28  15:07:19", " 2011-06-28  15:07:22", " 2011-06-28  15:07:24", " 2011-06-28  15:07:27", " 2011-06-28  15:07:30", " 2011-06-28  15:07:33", " 2011-06-28  15:07:36", " 2011-06-28  15:07:39", " 2011-06-28  15:07:41", " 2011-06-28  15:07:44", " 2011-06-28  15:07:47", " 2011-06-28  15:07:50", " 2011-06-28  15:07:53"], [" 802.00", " 802.00", " 802.00", " 802.00", " 802.00", " 802.00", " 802.00", " 802.00", " 802.00", " 802.00", " 802.00", " 802.00", " 802.00", " 802.00", " 802.00", " 802.00", " 802.00", " 802.00", " 802.00", " 802.00", " 802.00", " 802.00", " 802.00", " 802.00", " 802.00", " 802.00", " 802.00", " 802.00", " 802.00", " 802.00", " 802.00", " 802.00", " 802.00", " 802.00", " 802.00", " 802.00", " 802.00", " 802.00", " 802.00", " 802.00", " 802.00", " 802.00", " 802.00", " 802.00", " 802.00", " 802.00", " 802.00", " 802.00", " 802.00", " 802.00", " 802.00", " 802.00", " 802.00", " 802.00", " 802.00", " 802.00", " 802.00", " 802.00", " 802.00", " 802.00", " 802.00", " 802.00", " 802.00", " 802.00", " 802.00", " 802.00", " 802.00", " 802.00", " 802.00", " 802.00", " 802.00", " 802.00", " 802.00", " 802.00", " 802.00", " 802.00", " 802.00", " 802.00", " 802.00", " 802.00", " 802.00"], [" 4.00", " 4.10", " 4.20", " 4.30", " 4.40", " 4.50", " 4.60", " 4.70", " 4.80", " 4.90", " 5.00", " 5.10", " 5.20", " 5.30", " 5.40", " 5.50", " 5.60", " 5.70", " 5.80", " 5.90", " 6.00", " 6.10", " 6.20", " 6.30", " 6.40", " 6.50", " 6.60", " 6.70", " 6.80", " 6.90", " 7.00", " 7.10", " 7.20", " 7.30", " 7.40", " 7.50", " 7.60", " 7.70", " 7.80", " 7.90", " 8.00", " 8.10", " 8.20", " 8.30", " 8.40", " 8.50", " 8.60", " 8.70", " 8.80", " 8.90", " 9.00", " 9.10", " 9.20", " 9.30", " 9.40", " 9.50", " 9.60", " 9.70", " 9.80", " 9.90", " 10.00", " 10.10", " 10.20", " 10.30", " 10.40", " 10.50", " 10.60", " 10.70", " 10.80", " 10.90", " 11.00", " 11.10", " 11.20", " 11.30", " 11.40", " 11.50", " 11.60", " 11.70", " 11.80", " 11.90", " 12.00"], [" 0.04", " 0.04", " 0.04", " 0.04", " 0.04", " 0.04", " 0.04", " 0.04", " 0.04", " 0.04", " 0.04", " 0.04", " 0.04", " 0.04", " 0.04", " 0.04", " 0.04", " 0.04", " 0.04", " 0.04", " 0.04", " 0.04", " 0.04", " 0.04", " 0.04", " 0.04", " 0.04", " 0.04", " 0.04", " 0.04", " 0.04", " 0.04", " 0.04", " 0.04", " 0.04", " 0.04", " 0.04", " 0.04", " 0.04", " 0.04", " 0.04", " 0.04", " 0.04", " 0.04", " 0.04", " 0.04", " 0.04", " 0.04", " 0.04", " 0.04", " 0.04", " 0.04", " 0.04", " 0.04", " 0.04", " 0.04", " 0.04", " 0.04", " 0.04", " 0.04", " 0.04", " 0.04", " 0.04", " 0.04", " 0.04", " 0.04", " 0.04", " 0.04", " 0.04", " 0.04", " 0.04", " 0.04", " 0.04", " 0.04", " 0.04", " 0.04", " 0.04", " 0.04", " 0.04", " 0.04", " 0.04"], [" 0", " 0", " 0", " 0", " 0", " 0", " 0", " 0", " 0", " 0", " 0", " 0", " 0", " 0", " 0", " 0", " 0", " 0", " 0", " 0", " 0", " 0", " 0", " 0", " 0", " 0", " 0", " 0", " 0", " 0", " 0", " 0", " 0", " 0", " 0", " 0", " 0", " 0", " 0", " 0", " 0", " 0", " 0", " 0", " 0", " 0", " 0", " 0", " 0", " 0", " 0", " 0", " 0", " 0", " 0", " 0", " 0", " 0", " 0", " 0", " 0", " 0", " 0", " 0", " 0", " 0", " 0", " 0", " 0", " 0", " 0", " 0", " 0", " 0", " 0", " 0", " 0", " 0", " 0", " 0", " 0"], [" 0", " 0", " 0", " 0", " 0", " 0", " 0", " 0", " 0", " 0", " 0", " 0", " 0", " 0", " 0", " 0", " 0", " 0", " 0", " 0", " 0", " 0", " 0", " 0", " 0", " 0", " 0", " 0", " 0", " 0", " 0", " 0", " 0", " 0", " 0", " 0", " 0", " 0", " 0", " 0", " 0", " 0", " 0", " 0", " 0", " 0", " 0", " 0", " 0", " 0", " 0", " 0", " 0", " 0", " 0", " 0", " 0", " 0", " 0", " 0", " 0", " 0", " 0", " 0", " 0", " 0", " 0", " 0", " 0", " 0", " 0", " 0", " 0", " 0", " 0", " 0", " 0", " 0", " 0", " 0", " 0"], [" 404.6", " 398.5", " 375.5", " 422.3", " 379.5", " 343.2", " 393.3", " 392.2", " 368.9", " 424.4", " 372.7", " 318.8", " 349.7", " 310.0", " 253.3", " 253.5", " 233.3", " 215.8", " 252.2", " 260.6", " 219.4", " 213.5", " 204.7", " 211.9", " 236.0", " 230.9", " 210.6", " 214.9", " 215.9", " 227.9", " 237.4", " 214.6", " 199.6", " 215.6", " 255.9", " 235.4", " 229.8", " 238.3", " 218.6", " 244.5", " 277.4", " 245.4", " 241.5", " 248.4", " 245.5", " 269.8", " 270.8", " 254.3", " 255.2", " 255.7", " 274.8", " 277.4", " 244.4", " 237.4", " 253.0", " 243.3", " 246.6", " 259.4", " 227.7", " 219.8", " 237.8", " 228.4", " 217.3", " 209.6", " 207.2", " 203.9", " 212.1", " 209.4", " 203.7", " 222.7", " 222.8", " 219.9", " 238.4", " 234.6", " 243.7", " 259.6", " 267.7", " 270.1", " 260.8", " 263.5", " 270.9"], ["", "", "", "", "", "", "", "", "", "", "", "", "", "", "", "", "", "", "", "", "", "", "", "", "", "", "", "", "", "", "", "", "", "", "", "", "", "", "", "", "", "", "", "", "", "", "", "", "", "", "", "", "", "", "", "", "", "", "", "", "", "", "", "", "", "", "", "", "", "", "", "", "", "", "", "", "", "", "", "", ""], [" -1.580E+1", " -1.583E+1", " -1.570E+1", " -1.554E+1", " -1.594E+1", " -1.656E+1", " -1.648E+1", " -1.624E+1", " -1.643E+1", " -1.618E+1", " -1.663E+1", " -1.700E+1", " -1.686E+1", " -1.740E+1", " -1.730E+1", " -1.715E+1", " -1.716E+1", " -1.762E+1", " -1.784E+1", " -1.738E+1", " -1.777E+1", " -1.749E+1", " -1.757E+1", " -1.773E+1", " -1.730E+1", " -1.747E+1", " -1.778E+1", " -1.798E+1", " -1.791E+1", " -1.735E+1", " -1.720E+1", " -1.699E+1", " -1.741E+1", " -1.796E+1", " -1.780E+1", " -1.814E+1", " -1.765E+1", " -1.752E+1", " -1.784E+1", " -1.767E+1", " -1.793E+1", " -1.808E+1", " -1.790E+1", " -1.764E+1", " -1.741E+1", " -1.747E+1", " -1.696E+1", " -1.670E+1", " -1.693E+1", " -1.689E+1", " -1.684E+1", " -1.686E+1", " -1.689E+1", " -1.684E+1", " -1.682E+1", " -1.768E+1", " -1.760E+1", " -1.675E+1", " -1.707E+1", " -1.697E+1", " -1.684E+1", " -1.705E+1", " -1.666E+1", " -1.691E+1", " -1.670E+1", " -1.671E+1", " -1.721E+1", " -1.683E+1", " -1.724E+1", " -1.704E+1", " -1.739E+1", " -1.790E+1", " -1.771E+1", " -1.765E+1", " -1.715E+1", " -1.744E+1", " -1.805E+1", " -1.864E+1", " -1.878E+1", " -1.902E+1", " -1.834E+1"], [" -1.740E+1 ", " -1.745E+1 ", " -1.739E+1 ", " -1.710E+1 ", " -1.762E+1 ", " -1.835E+1 ", " -1.812E+1 ", " -1.788E+1 ", " -1.814E+1 ", " -1.773E+1 ", " -1.833E+1 ", " -1.888E+1 ", " -1.864E+1 ", " -1.932E+1 ", " -1.947E+1 ", " -1.932E+1 ", " -1.944E+1 ", " -2.000E+1 ", " -2.002E+1 ", " -1.951E+1 ", " -2.013E+1 ", " -1.989E+1 ", " -2.002E+1 ", " -2.013E+1 ", " -1.956E+1 ", " -1.976E+1 ", " -2.019E+1 ", " -2.037E+1 ", " -2.029E+1 ", " -1.966E+1 ", " -1.945E+1 ", " -1.938E+1 ", " -1.990E+1 ", " -2.034E+1 ", " -1.996E+1 ", " -2.040E+1 ", " -1.995E+1 ", " -1.977E+1 ", " -2.020E+1 ", " -1.989E+1 ", " -1.998E+1 ", " -2.029E+1 ", " -2.013E+1 ", " -1.983E+1 ", " -1.962E+1 ", " -1.956E+1 ", " -1.904E+1 ", " -1.886E+1 ", " -1.909E+1 ", " -1.905E+1 ", " -1.891E+1 ", " -1.891E+1 ", " -1.910E+1 ", " -1.909E+1 ", " -1.899E+1 ", " -1.990E+1 ", " -1.981E+1 ", " -1.889E+1 ", " -1.938E+1 ", " -1.932E+1 ", " -1.909E+1 ", " -1.935E+1 ", " -1.903E+1 ", " -1.933E+1 ", " -1.913E+1 ", " -1.917E+1 ", " -1.962E+1 ", " -1.925E+1 ", " -1.969E+1 ", " -1.938E+1 ", " -1.973E+1 ", " -2.025E+1 ", " -1.996E+1 ", " -1.992E+1 ", " -1.937E+1 ", " -1.958E+1 ", " -2.015E+1 ", " -2.073E+1 ", " -2.091E+1 ", " -2.114E+1 ", " -2.042E+1 "]]
  out "配列":dbl[][](array[numeric])=[[4.0, 4.1, 4.2, 4.3, 4.4, 4.5, 4.6, 4.7, 4.8, 4.9, 5.0, 5.1, 5.2, 5.3, 5.4, 5.5, 5.6, 5.7, 5.8, 5.9, 6.0, 6.1, 6.2, 6.3, 6.4, 6.5, 6.6, 6.7, 6.8, 6.9, 7.0, 7.1, 7.2, 7.3, 7.4, 7.5, 7.6, 7.7, 7.8, 7.9, 8.0, 8.1, 8.2, 8.3, 8.4, 8.5, 8.6, 8.7, 8.8, 8.9, 9.0, 9.1, 9.2, 9.3, 9.4, 9.5, 9.6, 9.7, 9.8, 9.9, 10.0, 10.1, 10.2, 10.3, 10.4, 10.5, 10.6, 10.7, 10.8, 10.9, 11.0, 11.1, 11.2, 11.3, 11.4, 11.5, 11.6, 11.7, 11.8, 11.9, 12.0], [-15.8, -15.83, -15.7, -15.54, -15.94, -16.56, -16.48, -16.24, -16.43, -16.18, -16.63, -17.0, -16.86, -17.4, -17.3, -17.15, -17.16, -17.62, -17.84, -17.38, -17.77, -17.49, -17.57, -17.73, -17.3, -17.47, -17.78, -17.98, -17.91, -17.35, -17.2, -16.99, -17.41, -17.96, -17.8, -18.14, -17.65, -17.52, -17.84, -17.67, -17.93, -18.08, -17.9, -17.64, -17.41, -17.47, -16.96, -16.7, -16.93, -16.89, -16.84, -16.86, -16.89, -16.84, -16.82, -17.68, -17.6, -16.75, -17.07, -16.97, -16.84, -17.05, -16.66, -16.91, -16.7, -16.71, -17.21, -16.83, -17.24, -17.04, -17.39, -17.9, -17.71, -17.65, -17.15, -17.44, -18.05, -18.64, -18.78, -19.02, -18.34], [-17.4, -17.45, -17.39, -17.1, -17.62, -18.35, -18.12, -17.88, -18.14, -17.73, -18.33, -18.88, -18.64, -19.32, -19.47, -19.32, -19.44, -20.0, -20.02, -19.51, -20.13, -19.89, -20.02, -20.13, -19.56, -19.76, -20.19, -20.37, -20.29, -19.66, -19.45, -19.38, -19.9, -20.34, -19.96, -20.4, -19.95, -19.77, -20.2, -19.89, -19.98, -20.29, -20.13, -19.83, -19.62, -19.56, -19.04, -18.86, -19.09, -19.05, -18.91, -18.91, -19.1, -19.09, -18.99, -19.9, -19.81, -18.89, -19.38, -19.32, -19.09, -19.35, -19.03, -19.33, -19.13, -19.17, -19.62, -19.25, -19.69, -19.38, -19.73, -20.25, -19.96, -19.92, -19.37, -19.58, -20.15, -20.73, -20.91, -21.14, -20.42], [-18.02, -18.32, -18.1, -18.06, -18.02, -18.44, -18.75, -18.42, -18.36, -18.56, -18.69, -18.5, -18.64, -18.83, -18.27, -18.42, -18.59, -18.67, -18.81, -18.43, -18.52, -18.3, -18.55, -18.78, -18.49, -18.49, -18.6, -18.49, -18.57, -18.3, -18.15, -17.75, -18.05, -18.46, -18.23, -18.46, -18.39, -18.41, -18.53, -18.69, -18.91, -18.8, -18.82, -18.94, -18.83, -19.07, -19.07, -18.88, -19.04, -18.93, -19.23, -19.43, -19.14, -19.22, -19.22, -19.7, -19.58, -19.29, -19.4, -19.26, -19.45, -19.49, -19.16, -19.41, -19.02, -19.43, -19.78, -19.41, -19.82, -19.45, -19.82, -20.16, -20.26, -20.29, -19.56, -19.53, -19.7, -19.97, -20.1, -19.97, -19.71], [-35.52, -36.15, -36.25, -35.83, -35.68, -36.61, -37.08, -36.11, -36.2, -36.94, -36.76, -36.21, -36.81, -37.21, -36.31, -36.3, -36.83, -37.16, -36.82, -36.5, -36.97, -36.79, -36.65, -37.09, -37.21, -37.03, -36.85, -36.99, -37.1, -36.94, -36.61, -36.39, -36.75, -37.01, -36.7, -37.11, -36.88, -36.85, -36.96, -37.31, -37.4, -37.2, -37.46, -37.4, -37.41, -37.74, -37.47, -37.19, -37.47, -37.34, -37.62, -37.69, -37.57, -37.72, -37.49, -38.11, -37.85, -37.6, -37.63, -37.54, -37.79, -37.66, -37.45, -37.91, -37.39, -37.52, -38.08, -37.58, -37.8, -37.52, -38.15, -38.46, -38.34, -38.2, -37.81, -37.81, -37.78, -38.0, -38.18, -38.08, -37.94], [-0.7584866783387779, -0.7724327798647377, -0.7737440826085024, -0.7828828756794595, -0.7888685720823426, -0.8065345719171537, -0.8166667399979259, -0.8219300891812409, -0.8361766477077268, -0.8474303946080284, -0.8554309765142929, -0.8657890985755239, -0.8707493863767344, -0.8831162055764202, -0.8998377819951561, -0.900522155832352, -0.9150871253398222, -0.9244671905020112, -0.9290788460513937, -0.9396587103543041, -0.9563465941376474, -0.9617296961695446, -0.9728355162077676, -0.9826759729593989, -0.9909304192974655, -0.9992080871115655, -1.005633074268317, -1.0120089152499685, -1.0208486830299932, -1.0360001058690196, -1.0407694532100713, -1.0443744123721266, -1.056561810129114, -1.0621521057134604, -1.0729699619917479, -1.080006016355919, -1.0880160901945968, -1.0963124662696209, -1.1028284055867907, -1.1139513537041563, -1.124893314192167, -1.1252502190715352, -1.136823269368949, -1.1402905139447546, -1.1527936074801661, -1.159785873737935, -1.1709555559753178, -1.1721132435387454, -1.1840425275302415, -1.1859791927079861, -1.201596270539345, -1.206031084031497, -1.2147749921850115, -1.2120076593479858, -1.2215366625554642, -1.2396254572546055, -1.2421375866352582, -1.2548587388090102, -1.261970626228731, -1.2597494045645459, -1.2719286737557132, -1.275327186374512, -1.2856910175115008, -1.3106501047801058, -1.325498345466935, -1.3321072776506147, -1.328720556493847, -1.3209202161010987, -1.3202540256005681, -1.341549381830708, -1.376275049260354, -1.3902644055867917, -1.3995032905175657, -1.3827304838700119, -1.3915387049045536, -1.3878590450380377, -1.3826059425468715, -1.3996233024956117, -1.4121663141921663, -1.406446722149381, -1.408545220449345], [26.875132875175, 26.863065947539578, 26.744103844529878, 26.56971078890642, 26.621346255694572, 26.541884544545436, 26.277356816077393, 26.255741447439576, 26.370329461099136, 26.330553259553916, 26.331650168744492, 26.41285009600213, 26.312084945739535, 26.304729926146507, 26.372729039978665, 26.285419962888064, 26.16262424379801, 26.340782228271742, 26.404840964095495, 26.279933703711933, 26.29130278561746, 26.43069811203212, 26.354475715238117, 26.31334972154937, 26.4303088711601, 26.411955353378225, 26.379677807506834, 26.48503002644503, 26.446781588479745, 26.26608784328541, 26.347990951058172, 26.418149899627398, 26.239447653725637, 26.193153405705313, 26.25313197093269, 26.106456247249938, 25.995906440809794, 26.029013301703003, 25.914300482232942, 25.773855219745624, 25.772526860374676, 25.633051633147407, 25.38188356511626, 25.31665307614243, 25.214492440498677, 24.98847603917124, 24.80855158470188, 24.682109709549103, 24.582621293362074, 24.589360765276265, 24.5563276166137, 24.488641801743743, 24.515475450047038, 24.585609487099713, 24.712311575886872, 24.70054250657422, 24.658751714926996, 24.632860034000753, 24.680907893508742, 24.662019846218804, 24.700034165796275, 24.61051086764891, 24.518307286828595, 24.55975456973118, 24.57080112069157, 24.37885742616503, 24.290265462565834, 24.358663506151988, 24.41328423031623, 24.43220176248361, 24.360485893760604, 24.244142338940865, 24.211347518092996, 24.355028818492265, 24.40407788039734, 24.453447594390987, 24.491819926665038, 24.503725585235227, 24.508389505100116, 24.57837639125314, 24.62991109646881], [26.875132875175, 26.863065947539578, 26.744103844529878, 26.56971078890642, 26.621346255694572, 26.541884544545436, 26.277356816077393, 26.255741447439576, 26.370329461099136, 26.330553259553916, 26.331650168744492, 26.41285009600213, 26.312084945739535, 26.304729926146507, 26.372729039978665, 26.285419962888064, 26.16262424379801, 26.340782228271742, 26.404840964095495, 26.279933703711933, 26.29130278561746, 26.43069811203212, 26.354475715238117, 26.31334972154937, 26.4303088711601, 26.411955353378225, 26.379677807506834, 26.48503002644503, 26.446781588479745, 26.26608784328541, 26.347990951058172, 26.418149899627398, 26.239447653725637, 26.193153405705313, 26.25313197093269, 26.106456247249938, 25.995906440809794, 26.029013301703003, 25.914300482232942, 25.773855219745624, 25.772526860374676, 25.633051633147407, 25.38188356511626, 25.31665307614243, 25.214492440498677, 24.98847603917124, 24.80855158470188, 24.682109709549103, 24.582621293362074, 24.589360765276265, 24.5563276166137, 24.488641801743743, 24.515475450047038, 24.585609487099713, 24.712311575886872, 24.70054250657422, 24.658751714926996, 24.632860034000753, 24.680907893508742, 24.662019846218804, 24.700034165796275, 24.61051086764891, 24.518307286828595, 24.55975456973118, 24.57080112069157, 24.37885742616503, 24.290265462565834, 24.358663506151988, 24.41328423031623, 24.43220176248361, 24.360485893760604, 24.244142338940865, 24.211347518092996, 24.355028818492265, 24.40407788039734, 24.453447594390987, 24.491819926665038, 24.503725585235227, 24.508389505100116, 24.57837639125314, 24.62991109646881], [21.79, 21.78041282831954, 21.772016700415026, 21.764580572510507, 21.75787340083005, 21.751664141597715, 21.745721751037564, 21.739815185373654, 21.73371340083005, 21.727185353630812, 21.72, 21.712015131182426, 21.703443878505908, 21.694588208319015, 21.685750086970312, 21.677231480808373, 21.669334356181764, 21.662360679439054, 21.65661241692881, 21.6523915349996, 21.65, 21.64963664695075, 21.65108778556134, 21.654036594213434, 21.658166251288694, 21.663159935168785, 21.668700824235376, 21.674472096870126, 21.680156931454704, 21.685438506370776, 21.69, 21.693608281014566, 21.696364979248727, 21.69845541482725, 21.70006490787491, 21.70137877851648, 21.702582346876735, 21.703860933080442, 21.705399857252374, 21.707384439517302, 21.71, 21.713380228990985, 21.71745229744376, 21.72209174647757, 21.727174117211664, 21.732574950765287, 21.738169788257686, 21.74383417080811, 21.74944363953581, 21.75487373556002, 21.76, 21.764660803021492, 21.768545830976237, 21.77130759926247, 21.772598623278437, 21.772071418422374, 21.76937850009252, 21.764172383687118, 21.756105584604406, 21.74483061824262, 21.73, 21.711516558923048, 21.6902843786513, 21.66745785647255, 21.64419138967459, 21.621639375545215, 21.600956211372228, 21.583296294443414, 21.569814022046575, 21.561663791469506, 21.56, 21.56554296128631, 21.577276654418565, 21.59375097484734, 21.61351581802321, 21.635121079396757, 21.657116654418566, 21.678052438539215, 21.69647832720928, 21.71094421587935, 21.72], [401.9140426735799, 394.75812785452376, 371.0614536288631, 416.7826185394593, 374.3243326980722, 340.4628582128464, 387.77874142440936, 387.77874142440936, 364.6516148294494, 420.62099002242826, 367.83744166083335, 315.7443592189742, 343.3659439767455, 305.51322405740643, 250.24981952690112, 250.24981952690044, 229.84356141214752, 212.96486468500444, 248.30775543404707, 258.20422615941976, 216.22344244475124, 209.76193734579428, 201.9891414146812, 209.76193734579485, 233.40282283656907, 228.08777292672426, 208.1809094089769, 211.35653207271164, 212.96486468500444, 224.62284785774372, 235.20671980907528, 211.35653207271164, 196.001465831908, 212.96486468500444, 252.21024001848184, 233.40282283656907, 226.34760271499096, 235.20671980907528, 216.22344244475124, 240.71810018385082, 275.0632414827429, 242.5892088875253, 238.86413487820636, 246.3837961976696, 242.5892088875253, 266.4693030754984, 268.58621557379115, 252.21024001848184, 252.21024001848184, 252.21024001848184, 270.7239727210061, 275.0632414827429, 242.5892088875253, 235.20671980907528, 250.24981952690112, 240.71810018385082, 242.58920888752598, 256.18717987357735, 224.62284785774372, 217.8740444657678, 235.20671980907528, 226.34760271499096, 214.5871091652999, 206.61327999467903, 205.05888360483368, 200.47347796194887, 208.1809094089769, 206.6132799946785, 201.98914141468066, 219.5390982463626, 219.5390982463626, 217.8740444657678, 235.20671980907528, 231.61517466578167, 240.71810018385014, 256.18717987357803, 264.3729373605166, 266.4693030754984, 258.2042261594205, 260.2406829166549, 268.5862155737904], [493.84895903214283, 433.24565278333415, 379.11058912875274, 440.9030761984687, 459.0423837532648, 372.7910986290328, 347.24464521462613, 450.61028235691697, 423.7200796186839, 337.0177122109987, 383.6913789782991, 442.34605016730944, 365.3733736554684, 332.26178028545655, 383.09854364283603, 407.73299354502177, 349.47585948123594, 311.6983152599363, 383.3094496837194, 373.1459282916804, 315.67898888407296, 309.9116996110668, 368.2457799526763, 336.70895345492414, 279.2101129321424, 304.71957660146904, 347.86738238453825, 311.9751112607674, 308.5040387984872, 293.819956182582, 319.9191052956271, 294.9361950317238, 287.0475308147238, 308.2263775429199, 319.9077692088333, 294.61243691347283, 317.3804969575367, 324.8051767984757, 326.4857413497107, 299.61170830774483, 318.4341606932475, 332.0434981680025, 298.2060435962275, 324.509483890819, 307.988080963883, 296.1069248148851, 335.6557985595628, 349.99012078132216, 332.8613515974338, 336.61479533358806, 340.3460068647048, 360.77533949445547, 335.6466782422743, 325.7511574259726, 360.43914597635114, 339.1367646034172, 359.9503789461819, 353.03649934533547, 364.11091909283124, 354.7065292788962, 343.40644826721217, 366.60946158027184, 345.04043241826685, 310.9891288004955, 326.43843479211074, 365.2885166198709, 330.45586648808364, 347.2453933763653, 374.51909936355645, 359.24989388389974, 320.19120992370824, 325.344025908027, 360.07715748061844, 389.42685209840624, 339.69975890794944, 338.39972075741883, 372.3055844056587, 383.48534508019736, 378.4175241715284, 375.9253887086987, 358.620920657038], [44091.32447076029, 43994.75831990658, 43910.363794247765, 43835.754925597816, 43768.5693795309, 43706.46383235776, 43647.11062298791, 43588.195660795885, 43527.41757468769, 43462.48809076271, 43391.13362632319, 43311.97790882033, 43227.17104451725, 43139.72567851012, 43052.631197314244, 42968.85292988594, 42891.33341788972, 42822.99572743096, 42766.74877891334, 42725.4946800432, 42702.13805924481, 42698.590543528124, 42712.760183244565, 42741.568408625026, 42781.945760703806, 42830.822369559966, 42885.120666639195, 42941.75032680826, 42997.60544836155, 43049.56398721866, 43094.48946500095, 43130.06033328056, 43157.25611739225, 43177.89050093843, 43193.784339969454, 43206.7632577428, 43218.65601368612, 43231.29365038, 43246.509420894174, 43266.13949825875, 43292.02446923266, 43325.500104797145, 43365.86189297414, 43411.89362514082, 43462.37641482925, 43516.0872568836, 43571.79793311995, 43628.27426628759, 43684.27572486647, 43738.55538169144, 43789.86022956885, 43836.55922049547, 43875.52363734714, 43903.24366145685, 43916.20778976079, 43910.913269789606, 43883.8793281495, 43831.663144010694, 43750.87848657975, 43638.21689725488, 43490.471253616546, 43307.0402806518, 43097.291831262795, 42872.93409664584, 42645.46253696376, 42426.13606749905, 42225.98364283205, 42055.840180019724, 41926.41091820634, 41848.36368056843, 41832.44907893275, 41885.49264450272, 41998.002230220256, 42156.481637149496, 42347.41014295894, 42557.11355843115, 42771.679781978426, 42976.91968141588, 43158.37470386311, 43301.37275969895, 43391.13362632319], [-42.304058133402506, -42.04170104561826, -42.25769085666673, -42.31033056902308, -42.699370793354305, -42.9673333159231, -42.837630586787604, -42.94984868225228, -43.07707400925531, -42.66207963493079, -42.98011802522254, -43.45648977225463, -43.280806658564245, -43.634589212892486, -44.018645325326226, -43.81372941546897, -43.76980228766497, -43.96918926175765, -43.986226970817, -44.024745724653854, -44.2990635530348, -44.094645933336906, -43.98832153150062, -43.946678895226086, -43.67736451771449, -43.85248156438922, -44.072831890236266, -44.26537276912129, -44.13913616205879, -44.009433614744594, -43.918231331259655, -44.030884167315875, -44.31466142206972, -44.493289418320245, -44.49089464719869, -44.7392295395062, -44.42057403155067, -44.2279010527397, -44.53456965048816, -44.33192110058992, -44.35971000898137, -44.75547143915319, -44.79102247770662, -44.468178244294656, -44.43278840023204, -44.46644883392027, -44.11964718633102, -44.16930583654094, -44.32129391903585, -44.37722482951502, -44.03954965889642, -43.91817166456329, -44.19873556734652, -43.99862590961723, -43.84111258473843, -44.21531647455938, -44.297269712777904, -43.75561086527098, -43.918462838542595, -43.99076991963976, -43.63530516028899, -43.90978604302725, -43.952711025560276, -43.90897239791697, -44.08618137809738, -43.893909627344996, -44.15642536559794, -44.10336227759402, -44.06279401495067, -44.20067317922716, -44.219315282199645, -44.486166112971304, -44.20807200459492, -43.97480625686816, -44.12732399906333, -44.380180854477324, -44.765220199391514, -45.03550740084957, -45.01000250395328, -45.301369374868585, -44.81874285356317], [-43.9040581334025, -43.66170104561826, -43.947690856666725, -43.87033056902308, -44.379370793354305, -44.757333315923105, -44.477630586787605, -44.58984868225228, -44.78707400925531, -44.21207963493079, -44.68011802522254, -45.33648977225463, -45.060806658564246, -45.55458921289249, -46.18864532532622, -45.98372941546897, -46.049802287664974, -46.34918926175765, -46.16622697081701, -46.15474572465385, -46.6590635530348, -46.49464593333691, -46.43832153150062, -46.34667889522608, -45.937364517714485, -46.14248156438922, -46.48283189023627, -46.65537276912129, -46.519136162058786, -46.3194336147446, -46.168231331259655, -46.420884167315876, -46.80466142206972, -46.87328941832025, -46.65089464719868, -46.999229539506196, -46.72057403155067, -46.4779010527397, -46.89456965048816, -46.55192110058992, -46.40971000898137, -46.96547143915319, -47.021022477706616, -46.65817824429465, -46.64278840023205, -46.55644883392027, -46.19964718633102, -46.32930583654094, -46.481293919035856, -46.537224829515026, -46.10954965889642, -45.968171664563286, -46.408735567346525, -46.24862590961723, -46.01111258473843, -46.43531647455938, -46.5072697127779, -45.89561086527098, -46.2284628385426, -46.34076991963976, -45.88530516028899, -46.20978604302725, -46.32271102556028, -46.32897239791697, -46.516181378097386, -46.353909627345, -46.56642536559794, -46.523362277594025, -46.51279401495067, -46.540673179227156, -46.55931528219965, -46.8361661129713, -46.45807200459492, -46.24480625686816, -46.347323999063335, -46.52018085447732, -46.865220199391516, -47.12550740084957, -47.14000250395328, -47.42136937486859, -46.89874285356318], [0.0, 0.0, 0.0, 0.0, 0.0, 0.0, 0.0, 0.0, 0.0, 0.0, 1.9830446790355936, 2.2573625074165378, 2.0413726963680716, 1.988732984011719, 1.6369839181040078, 1.6369839181040078, 1.6369839181040078, 1.6369839181040078, 1.6369839181040078, 1.6369839181040078, 1.3189455278122608, 1.0182568944705537, 1.0182568944705537, 0.6800722091772329, 0.8159249006057578, 0.8159249006057578, 1.0618650217917107, 1.0618650217917107, 1.0618650217917107, 1.0618650217917107, 1.0618650217917107, 1.0618650217917107, 1.0781069214387031, 1.113657959992132, 1.113657959992132, 0.9385409133173965, 0.8727911464469642, 0.8727911464469642, 0.8727911464469642, 0.8727911464469642, 0.8727911464469642, 0.7601383103907438, 0.8728508131433301, 0.8728508131433301, 0.8728508131433301, 0.9499098929681864, 0.9499098929681864, 0.9499098929681864, 1.035411612435638, 1.035411612435638, 1.035411612435638, 1.1557173174176256, 1.1557173174176256, 0.8328730840056622, 0.8311436736312743, 0.8311436736312743, 0.7419196692260286, 0.7419196692260286, 0.7419196692260286, 0.7419196692260286, 0.6619645524889108, 0.6619645524889108, 0.8508609526823108, 0.8508609526823108, 0.8508609526823108, 0.8508609526823108, 0.8508609526823108, 1.1299150391025208, 1.4002022405605743, 1.4002022405605743, 1.6660642145795919, 0.0, 0.0, 0.0, 0.0, 0.0, 0.0, 0.0, 0.0, 0.0, 0.0]]
  out "XYグラフ 6":cluster{"データ配列":dbl[], "データ配列":dbl[]}[](graph)=[{"データ配列"=[4.0, 4.1, 4.2, 4.3, 4.4, 4.5, 4.6, 4.7, 4.8, 4.9, 5.0, 5.1, 5.2, 5.3, 5.4, 5.5, 5.6, 5.7, 5.8, 5.9, 6.0, 6.1, 6.2, 6.3, 6.4, 6.5, 6.6, 6.7, 6.8, 6.9, 7.0, 7.1, 7.2, 7.3, 7.4, 7.5, 7.6, 7.7, 7.8, 7.9, 8.0, 8.1, 8.2, 8.3, 8.4, 8.5, 8.6, 8.7, 8.8, 8.9, 9.0, 9.1, 9.2, 9.3, 9.4, 9.5, 9.6, 9.7, 9.8, 9.9, 10.0, 10.1, 10.2, 10.3, 10.4, 10.5, 10.6, 10.7, 10.8, 10.9, 11.0, 11.1, 11.2, 11.3, 11.4, 11.5, 11.6, 11.7, 11.8, 11.9, 12.0], "データ配列"=[-15.8, -15.83, -15.7, -15.54, -15.94, -16.56, -16.48, -16.24, -16.43, -16.18, -16.63, -17.0, -16.86, -17.4, -17.3, -17.15, -17.16, -17.62, -17.84, -17.38, -17.77, -17.49, -17.57, -17.73, -17.3, -17.47, -17.78, -17.98, -17.91, -17.35, -17.2, -16.99, -17.41, -17.96, -17.8, -18.14, -17.65, -17.52, -17.84, -17.67, -17.93, -18.08, -17.9, -17.64, -17.41, -17.47, -16.96, -16.7, -16.93, -16.89, -16.84, -16.86, -16.89, -16.84, -16.82, -17.68, -17.6, -16.75, -17.07, -16.97, -16.84, -17.05, -16.66, -16.91, -16.7, -16.71, -17.21, -16.83, -17.24, -17.04, -17.39, -17.9, -17.71, -17.65, -17.15, -17.44, -18.05, -18.64, -18.78, -19.02, -18.34]}, {"データ配列"=[4.0, 4.1, 4.2, 4.3, 4.4, 4.5, 4.6, 4.7, 4.8, 4.9, 5.0, 5.1, 5.2, 5.3, 5.4, 5.5, 5.6, 5.7, 5.8, 5.9, 6.0, 6.1, 6.2, 6.3, 6.4, 6.5, 6.6, 6.7, 6.8, 6.9, 7.0, 7.1, 7.2, 7.3, 7.4, 7.5, 7.6, 7.7, 7.8, 7.9, 8.0, 8.1, 8.2, 8.3, 8.4, 8.5, 8.6, 8.7, 8.8, 8.9, 9.0, 9.1, 9.2, 9.3, 9.4, 9.5, 9.6, 9.7, 9.8, 9.9, 10.0, 10.1, 10.2, 10.3, 10.4, 10.5, 10.6, 10.7, 10.8, 10.9, 11.0, 11.1, 11.2, 11.3, 11.4, 11.5, 11.6, 11.7, 11.8, 11.9, 12.0], "データ配列"=[-17.4, -17.45, -17.39, -17.1, -17.62, -18.35, -18.12, -17.88, -18.14, -17.73, -18.33, -18.88, -18.64, -19.32, -19.47, -19.32, -19.44, -20.0, -20.02, -19.51, -20.13, -19.89, -20.02, -20.13, -19.56, -19.76, -20.19, -20.37, -20.29, -19.66, -19.45, -19.38, -19.9, -20.34, -19.96, -20.4, -19.95, -19.77, -20.2, -19.89, -19.98, -20.29, -20.13, -19.83, -19.62, -19.56, -19.04, -18.86, -19.09, -19.05, -18.91, -18.91, -19.1, -19.09, -18.99, -19.9, -19.81, -18.89, -19.38, -19.32, -19.09, -19.35, -19.03, -19.33, -19.13, -19.17, -19.62, -19.25, -19.69, -19.38, -19.73, -20.25, -19.96, -19.92, -19.37, -19.58, -20.15, -20.73, -20.91, -21.14, -20.42]}, {"データ配列"=[4.0, 4.1, 4.2, 4.3, 4.4, 4.5, 4.6, 4.7, 4.8, 4.9, 5.0, 5.1, 5.2, 5.3, 5.4, 5.5, 5.6, 5.7, 5.8, 5.9, 6.0, 6.1, 6.2, 6.3, 6.4, 6.5, 6.6, 6.7, 6.8, 6.9, 7.0, 7.1, 7.2, 7.3, 7.4, 7.5, 7.6, 7.7, 7.8, 7.9, 8.0, 8.1, 8.2, 8.3, 8.4, 8.5, 8.6, 8.7, 8.8, 8.9, 9.0, 9.1, 9.2, 9.3, 9.4, 9.5, 9.6, 9.7, 9.8, 9.9, 10.0, 10.1, 10.2, 10.3, 10.4, 10.5, 10.6, 10.7, 10.8, 10.9, 11.0, 11.1, 11.2, 11.3, 11.4, 11.5, 11.6, 11.7, 11.8, 11.9, 12.0], "データ配列"=[-18.02, -18.32, -18.1, -18.06, -18.02, -18.44, -18.75, -18.42, -18.36, -18.56, -18.69, -18.5, -18.64, -18.83, -18.27, -18.42, -18.59, -18.67, -18.81, -18.43, -18.52, -18.3, -18.55, -18.78, -18.49, -18.49, -18.6, -18.49, -18.57, -18.3, -18.15, -17.75, -18.05, -18.46, -18.23, -18.46, -18.39, -18.41, -18.53, -18.69, -18.91, -18.8, -18.82, -18.94, -18.83, -19.07, -19.07, -18.88, -19.04, -18.93, -19.23, -19.43, -19.14, -19.22, -19.22, -19.7, -19.58, -19.29, -19.4, -19.26, -19.45, -19.49, -19.16, -19.41, -19.02, -19.43, -19.78, -19.41, -19.82, -19.45, -19.82, -20.16, -20.26, -20.29, -19.56, -19.53, -19.7, -19.97, -20.1, -19.97, -19.71]}, {"データ配列"=[4.0, 4.1, 4.2, 4.3, 4.4, 4.5, 4.6, 4.7, 4.8, 4.9, 5.0, 5.1, 5.2, 5.3, 5.4, 5.5, 5.6, 5.7, 5.8, 5.9, 6.0, 6.1, 6.2, 6.3, 6.4, 6.5, 6.6, 6.7, 6.8, 6.9, 7.0, 7.1, 7.2, 7.3, 7.4, 7.5, 7.6, 7.7, 7.8, 7.9, 8.0, 8.1, 8.2, 8.3, 8.4, 8.5, 8.6, 8.7, 8.8, 8.9, 9.0, 9.1, 9.2, 9.3, 9.4, 9.5, 9.6, 9.7, 9.8, 9.9, 10.0, 10.1, 10.2, 10.3, 10.4, 10.5, 10.6, 10.7, 10.8, 10.9, 11.0, 11.1, 11.2, 11.3, 11.4, 11.5, 11.6, 11.7, 11.8, 11.9, 12.0], "データ配列"=[-35.52, -36.15, -36.25, -35.83, -35.68, -36.61, -37.08, -36.11, -36.2, -36.94, -36.76, -36.21, -36.81, -37.21, -36.31, -36.3, -36.83, -37.16, -36.82, -36.5, -36.97, -36.79, -36.65, -37.09, -37.21, -37.03, -36.85, -36.99, -37.1, -36.94, -36.61, -36.39, -36.75, -37.01, -36.7, -37.11, -36.88, -36.85, -36.96, -37.31, -37.4, -37.2, -37.46, -37.4, -37.41, -37.74, -37.47, -37.19, -37.47, -37.34, -37.62, -37.69, -37.57, -37.72, -37.49, -38.11, -37.85, -37.6, -37.63, -37.54, -37.79, -37.66, -37.45, -37.91, -37.39, -37.52, -38.08, -37.58, -37.8, -37.52, -38.15, -38.46, -38.34, -38.2, -37.81, -37.81, -37.78, -38.0, -38.18, -38.08, -37.94]}, {"データ配列"=[4.0, 4.1, 4.2, 4.3, 4.4, 4.5, 4.6, 4.7, 4.8, 4.9, 5.0, 5.1, 5.2, 5.3, 5.4, 5.5, 5.6, 5.7, 5.8, 5.9, 6.0, 6.1, 6.2, 6.3, 6.4, 6.5, 6.6, 6.7, 6.8, 6.9, 7.0, 7.1, 7.2, 7.3, 7.4, 7.5, 7.6, 7.7, 7.8, 7.9, 8.0, 8.1, 8.2, 8.3, 8.4, 8.5, 8.6, 8.7, 8.8, 8.9, 9.0, 9.1, 9.2, 9.3, 9.4, 9.5, 9.6, 9.7, 9.8, 9.9, 10.0, 10.1, 10.2, 10.3, 10.4, 10.5, 10.6, 10.7, 10.8, 10.9, 11.0, 11.1, 11.2, 11.3, 11.4, 11.5, 11.6, 11.7, 11.8, 11.9, 12.0], "データ配列"=[-0.7584866783387779, -0.7724327798647377, -0.7737440826085024, -0.7828828756794595, -0.7888685720823426, -0.8065345719171537, -0.8166667399979259, -0.8219300891812409, -0.8361766477077268, -0.8474303946080284, -0.8554309765142929, -0.8657890985755239, -0.8707493863767344, -0.8831162055764202, -0.8998377819951561, -0.900522155832352, -0.9150871253398222, -0.9244671905020112, -0.9290788460513937, -0.9396587103543041, -0.9563465941376474, -0.9617296961695446, -0.9728355162077676, -0.9826759729593989, -0.9909304192974655, -0.9992080871115655, -1.005633074268317, -1.0120089152499685, -1.0208486830299932, -1.0360001058690196, -1.0407694532100713, -1.0443744123721266, -1.056561810129114, -1.0621521057134604, -1.0729699619917479, -1.080006016355919, -1.0880160901945968, -1.0963124662696209, -1.1028284055867907, -1.1139513537041563, -1.124893314192167, -1.1252502190715352, -1.136823269368949, -1.1402905139447546, -1.1527936074801661, -1.159785873737935, -1.1709555559753178, -1.1721132435387454, -1.1840425275302415, -1.1859791927079861, -1.201596270539345, -1.206031084031497, -1.2147749921850115, -1.2120076593479858, -1.2215366625554642, -1.2396254572546055, -1.2421375866352582, -1.2548587388090102, -1.261970626228731, -1.2597494045645459, -1.2719286737557132, -1.275327186374512, -1.2856910175115008, -1.3106501047801058, -1.325498345466935, -1.3321072776506147, -1.328720556493847, -1.3209202161010987, -1.3202540256005681, -1.341549381830708, -1.376275049260354, -1.3902644055867917, -1.3995032905175657, -1.3827304838700119, -1.3915387049045536, -1.3878590450380377, -1.3826059425468715, -1.3996233024956117, -1.4121663141921663, -1.406446722149381, -1.408545220449345]}, {"データ配列"=[4.0, 4.1, 4.2, 4.3, 4.4, 4.5, 4.6, 4.7, 4.8, 4.9, 5.0, 5.1, 5.2, 5.3, 5.4, 5.5, 5.6, 5.7, 5.8, 5.9, 6.0, 6.1, 6.2, 6.3, 6.4, 6.5, 6.6, 6.7, 6.8, 6.9, 7.0, 7.1, 7.2, 7.3, 7.4, 7.5, 7.6, 7.7, 7.8, 7.9, 8.0, 8.1, 8.2, 8.3, 8.4, 8.5, 8.6, 8.7, 8.8, 8.9, 9.0, 9.1, 9.2, 9.3, 9.4, 9.5, 9.6, 9.7, 9.8, 9.9, 10.0, 10.1, 10.2, 10.3, 10.4, 10.5, 10.6, 10.7, 10.8, 10.9, 11.0, 11.1, 11.2, 11.3, 11.4, 11.5, 11.6, 11.7, 11.8, 11.9, 12.0], "データ配列"=[26.875132875175, 26.863065947539578, 26.744103844529878, 26.56971078890642, 26.621346255694572, 26.541884544545436, 26.277356816077393, 26.255741447439576, 26.370329461099136, 26.330553259553916, 26.331650168744492, 26.41285009600213, 26.312084945739535, 26.304729926146507, 26.372729039978665, 26.285419962888064, 26.16262424379801, 26.340782228271742, 26.404840964095495, 26.279933703711933, 26.29130278561746, 26.43069811203212, 26.354475715238117, 26.31334972154937, 26.4303088711601, 26.411955353378225, 26.379677807506834, 26.48503002644503, 26.446781588479745, 26.26608784328541, 26.347990951058172, 26.418149899627398, 26.239447653725637, 26.193153405705313, 26.25313197093269, 26.106456247249938, 25.995906440809794, 26.029013301703003, 25.914300482232942, 25.773855219745624, 25.772526860374676, 25.633051633147407, 25.38188356511626, 25.31665307614243, 25.214492440498677, 24.98847603917124, 24.80855158470188, 24.682109709549103, 24.582621293362074, 24.589360765276265, 24.5563276166137, 24.488641801743743, 24.515475450047038, 24.585609487099713, 24.712311575886872, 24.70054250657422, 24.658751714926996, 24.632860034000753, 24.680907893508742, 24.662019846218804, 24.700034165796275, 24.61051086764891, 24.518307286828595, 24.55975456973118, 24.57080112069157, 24.37885742616503, 24.290265462565834, 24.358663506151988, 24.41328423031623, 24.43220176248361, 24.360485893760604, 24.244142338940865, 24.211347518092996, 24.355028818492265, 24.40407788039734, 24.453447594390987, 24.491819926665038, 24.503725585235227, 24.508389505100116, 24.57837639125314, 24.62991109646881]}, {"データ配列"=[4.0, 4.1, 4.2, 4.3, 4.4, 4.5, 4.6, 4.7, 4.8, 4.9, 5.0, 5.1, 5.2, 5.3, 5.4, 5.5, 5.6, 5.7, 5.8, 5.9, 6.0, 6.1, 6.2, 6.3, 6.4, 6.5, 6.6, 6.7, 6.8, 6.9, 7.0, 7.1, 7.2, 7.3, 7.4, 7.5, 7.6, 7.7, 7.8, 7.9, 8.0, 8.1, 8.2, 8.3, 8.4, 8.5, 8.6, 8.7, 8.8, 8.9, 9.0, 9.1, 9.2, 9.3, 9.4, 9.5, 9.6, 9.7, 9.8, 9.9, 10.0, 10.1, 10.2, 10.3, 10.4, 10.5, 10.6, 10.7, 10.8, 10.9, 11.0, 11.1, 11.2, 11.3, 11.4, 11.5, 11.6, 11.7, 11.8, 11.9, 12.0], "データ配列"=[21.79, 21.78041282831954, 21.772016700415026, 21.764580572510507, 21.75787340083005, 21.751664141597715, 21.745721751037564, 21.739815185373654, 21.73371340083005, 21.727185353630812, 21.72, 21.712015131182426, 21.703443878505908, 21.694588208319015, 21.685750086970312, 21.677231480808373, 21.669334356181764, 21.662360679439054, 21.65661241692881, 21.6523915349996, 21.65, 21.64963664695075, 21.65108778556134, 21.654036594213434, 21.658166251288694, 21.663159935168785, 21.668700824235376, 21.674472096870126, 21.680156931454704, 21.685438506370776, 21.69, 21.693608281014566, 21.696364979248727, 21.69845541482725, 21.70006490787491, 21.70137877851648, 21.702582346876735, 21.703860933080442, 21.705399857252374, 21.707384439517302, 21.71, 21.713380228990985, 21.71745229744376, 21.72209174647757, 21.727174117211664, 21.732574950765287, 21.738169788257686, 21.74383417080811, 21.74944363953581, 21.75487373556002, 21.76, 21.764660803021492, 21.768545830976237, 21.77130759926247, 21.772598623278437, 21.772071418422374, 21.76937850009252, 21.764172383687118, 21.756105584604406, 21.74483061824262, 21.73, 21.711516558923048, 21.6902843786513, 21.66745785647255, 21.64419138967459, 21.621639375545215, 21.600956211372228, 21.583296294443414, 21.569814022046575, 21.561663791469506, 21.56, 21.56554296128631, 21.577276654418565, 21.59375097484734, 21.61351581802321, 21.635121079396757, 21.657116654418566, 21.678052438539215, 21.69647832720928, 21.71094421587935, 21.72]}]
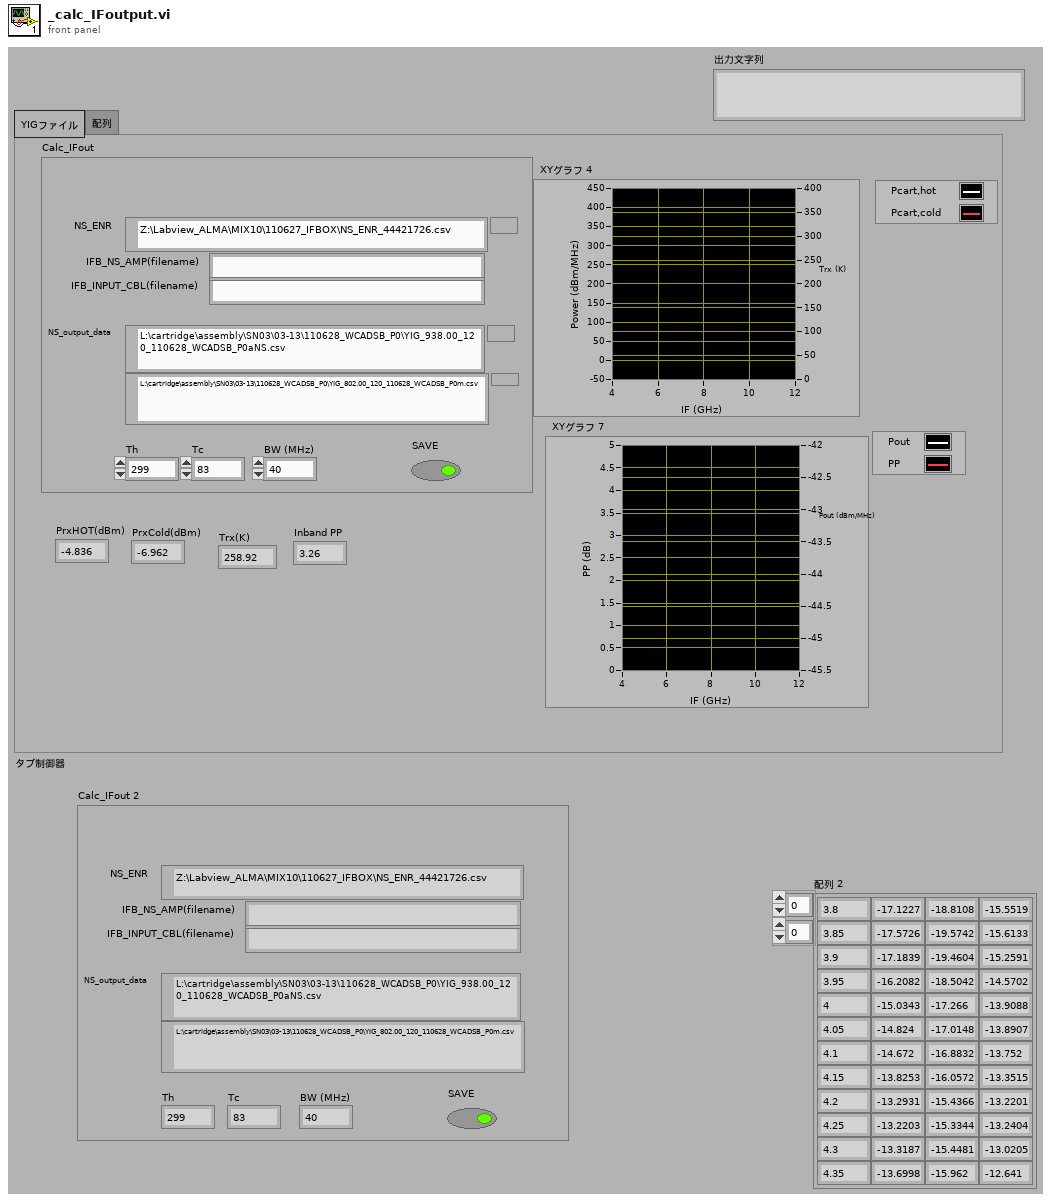
[diagram p1: front panel]
types:
  T1 = cluster{"Th":dbl, "Tc":dbl, "BW (MHz)":dbl, "NS_output_data":path, "Rx_output_data":path, "NS_ENR":path, "SAVE":bool, "IFB_NS_AMP(filename)":string, "IFB_INPUT_CBL(filename) ":string}
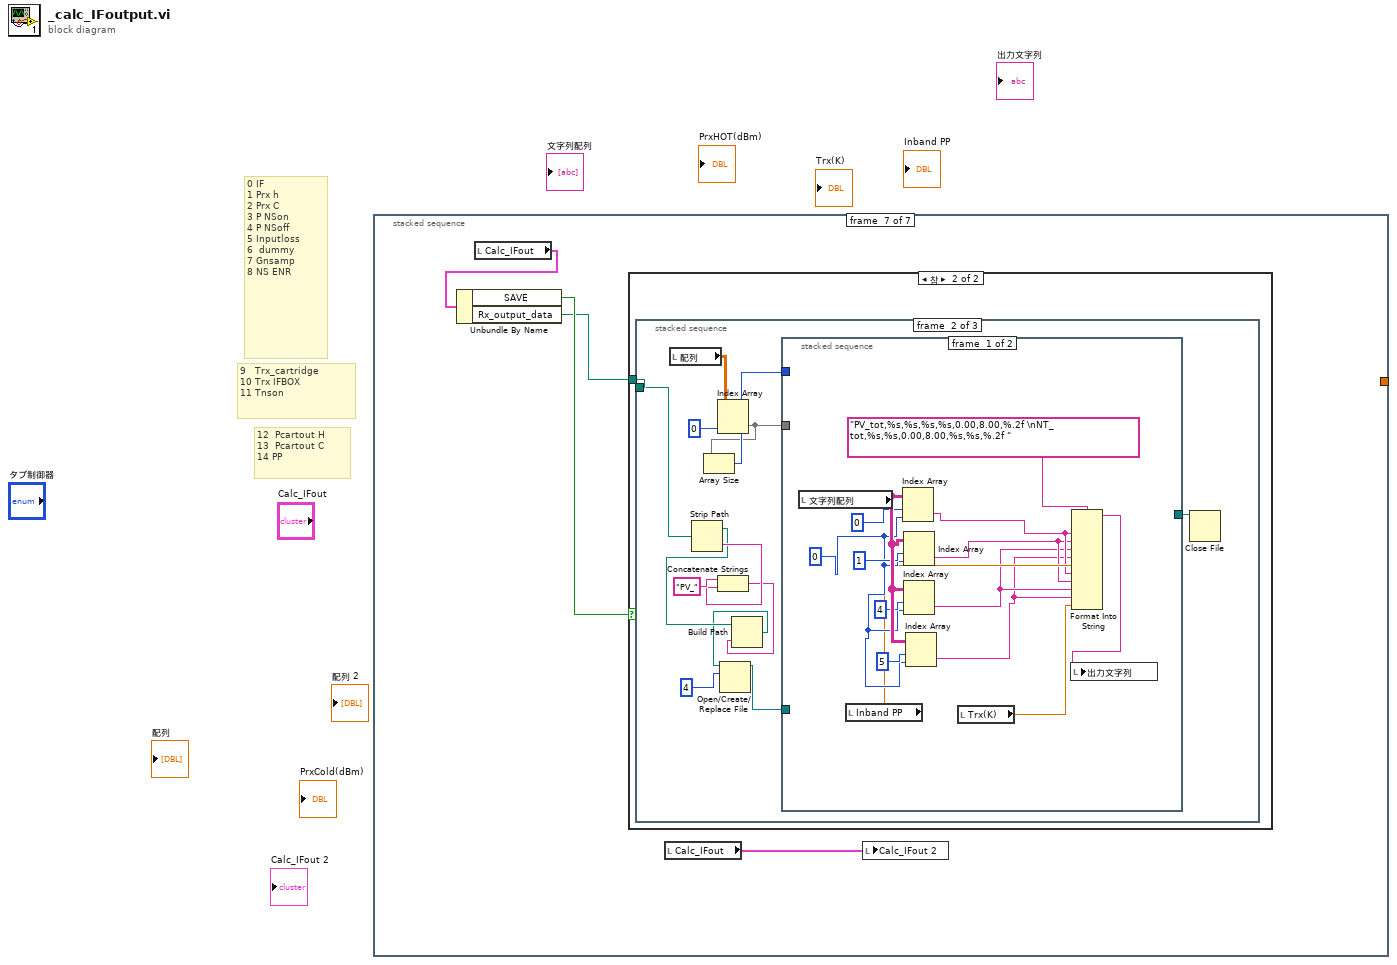
[diagram p0: block diagram]
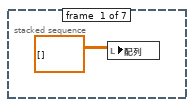
[diagram p2: hidden frame]
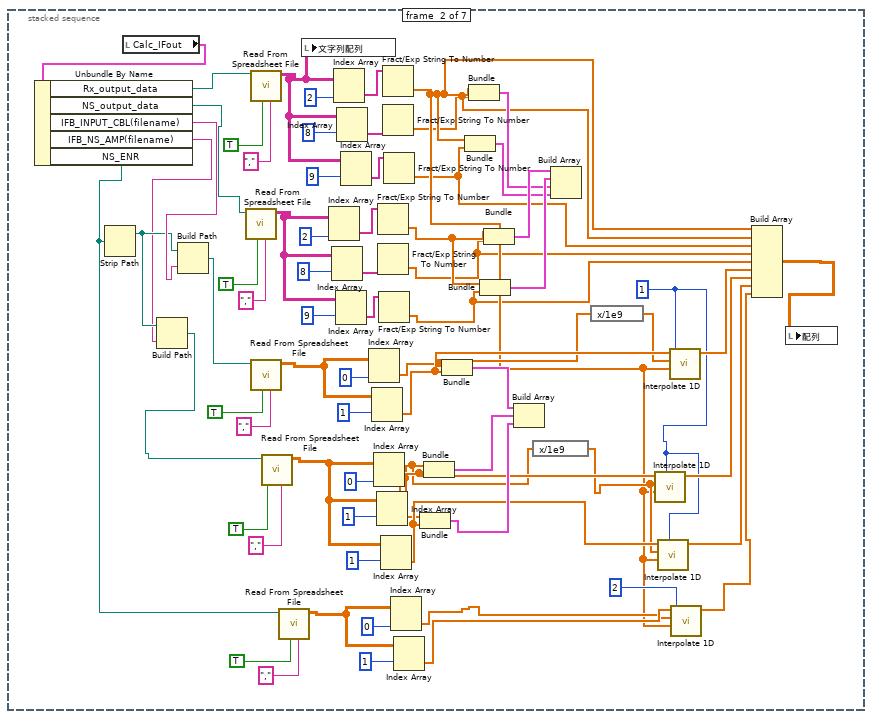
[diagram p3: hidden frame]
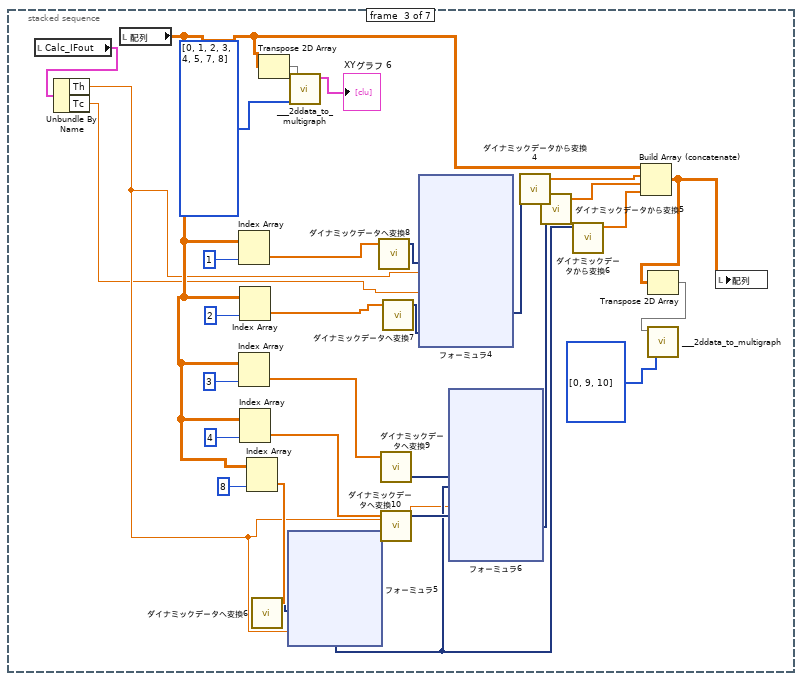
[diagram p4: hidden frame]
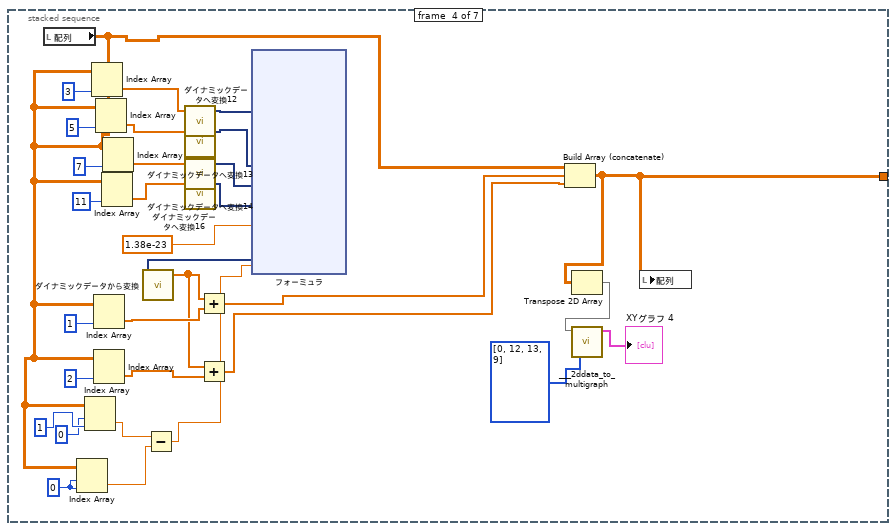
[diagram p5: hidden frame]
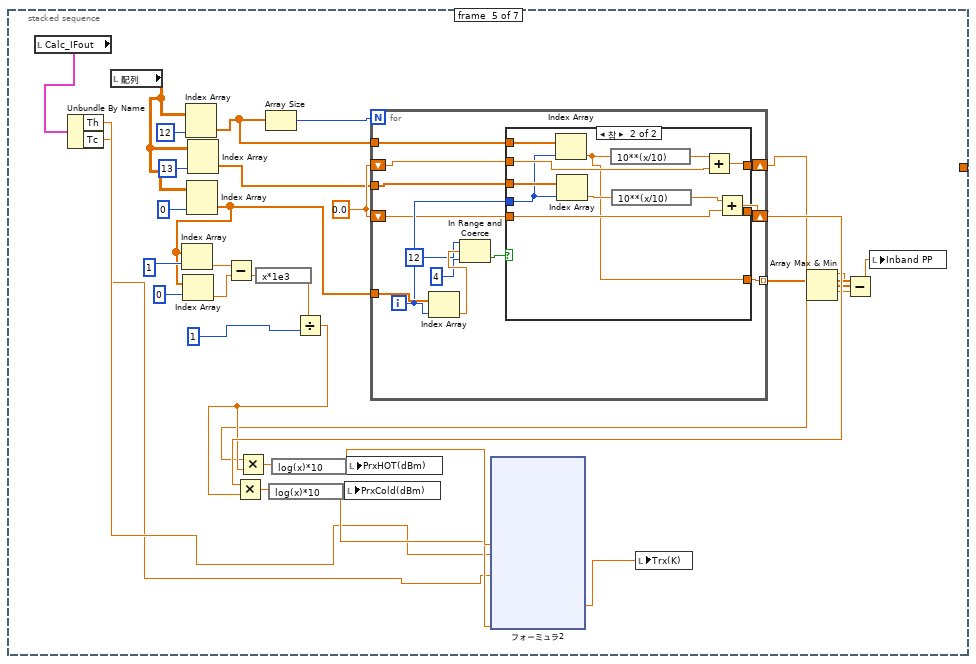
[diagram p6: hidden frame]
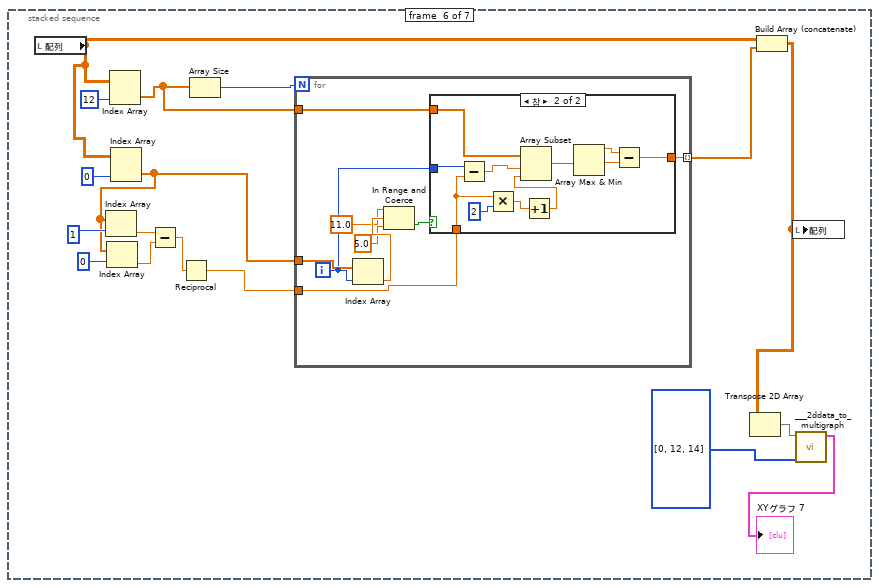
[diagram p8: hidden frame]
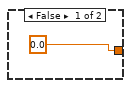
[diagram p9: hidden frame]
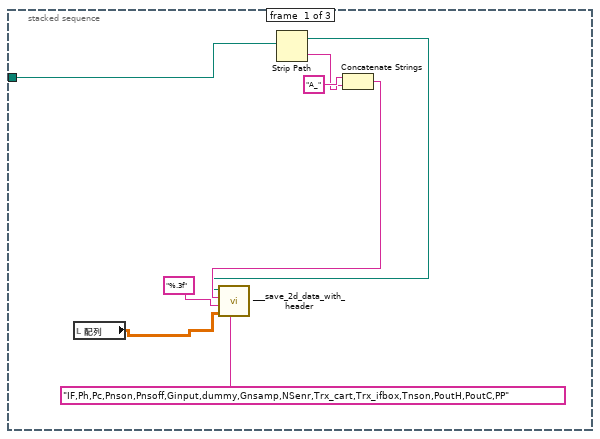
[diagram p11: hidden frame]
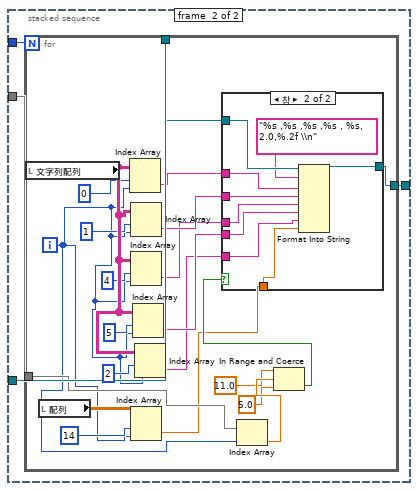
[diagram p12: hidden frame]
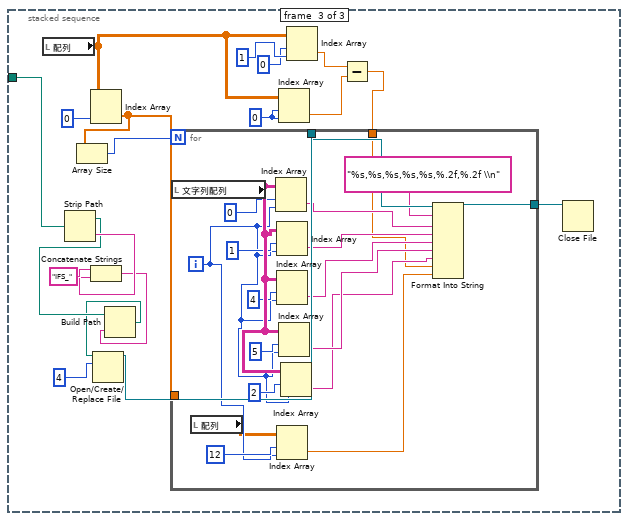
[diagram p14: hidden frame]
diagram:
  # "12  Pcartout H\n13  Pcartout C\n14 PP"
  # "9   Trx_cartridge\n10 Trx IFBOX\n11 Tnson"
  # "0 IF\n1 Prx h\n2 Prx C\n3 P NSon\n4 P NSoff\n5 Inputloss\n6  dummy\n7 Gnsamp\n8 NS ENR"
  n1 = stacked-sequence {
    tunnel: [_ _ _ w540 _ _ _] -> _
    frame #0 {
      n2 = local write "配列"(dbl[][] []) -> ()
    }
    frame #1 {
      w31 = 1
      n3 = local read "Calc_IFout"() -> (w8:T1)
      n4 = Unbundle By Name(w8) -> ("Rx_output_data"=w29:path, "NS_output_data"=w13:path, "IFB_INPUT_CBL(filename)"=w6:string, "IFB_NS_AMP(filename)"=w2:string, "NS_ENR"=w7:path)
      n5 = Strip Path(path=w7) -> (stripped path=w3:path)  [unwired: 1 out]
      n6 = Build Path(base path=w3, name or relative path=w2) -> (appended path=w4:path)
      n7 = Build Path(base path=w3, name or relative path=w6) -> (appended path=w5:path)
      n8 = call-poly <vilib>:"Read From Spreadsheet File.vi"("delimiter (\\t)"=",", "transpose (no:F)"=TRUE, "file path (dialog if empty)"=w13) -> ("all rows"=w19:string[][])  [unwired: 4 in, 4 out]
      n9 = call-poly <vilib>:"Read From Spreadsheet File.vi"("delimiter (\\t)"=",", "transpose (no:F)"=TRUE, "file path (dialog if empty)"=w29) -> ("all rows"=w9:string[][])  [unwired: 4 in, 4 out]
      n10 = call-poly <vilib>:"Read From Spreadsheet File.vi"("delimiter (\\t)"=",", "transpose (no:F)"=TRUE, "file path (dialog if empty)"=w5) -> ("all rows"=w54:dbl[][])  [unwired: 4 in, 4 out]
      n11 = call-poly <vilib>:"Read From Spreadsheet File.vi"("delimiter (\\t)"=",", "transpose (no:F)"=TRUE, "file path (dialog if empty)"=w4) -> ("all rows"=w59:dbl[][])  [unwired: 4 in, 4 out]
      n12 = call-poly <vilib>:"Read From Spreadsheet File.vi"("delimiter (\\t)"=",", "transpose (no:F)"=TRUE, "file path (dialog if empty)"=w7) -> ("all rows"=w44:dbl[][])  [unwired: 4 in, 4 out]
      n13 = local write "文字列配列"(w9) -> ()
      n14 = Index Array(array=w19, index (row)=2) -> (element=w20:string[])  [unwired: 1 in]
      n15 = Index Array(array=w19, index (row)=8) -> (element=w21:string[])  [unwired: 1 in]
      n16 = Index Array(array=w9, index (row)=2) -> (element=w28:string[])  [unwired: 1 in]
      n17 = Index Array(array=w19, index (row)=9) -> (element=w22:string[])  [unwired: 1 in]
      n18 = Index Array(array=w9, index (row)=8) -> (element=w26:string[])  [unwired: 1 in]
      n19 = Index Array(array=w9, index (row)=9) -> (element=w24:string[])  [unwired: 1 in]
      n20 = Index Array(array=w54, index (row)=0) -> (element=w36:dbl[])  [unwired: 1 in]
      n21 = Index Array(array=w54, index (row)=1) -> (element=w50:dbl[])  [unwired: 1 in]
      n22 = Index Array(array=w59, index (row)=0) -> (element=w34:dbl[])  [unwired: 1 in]
      n23 = Index Array(array=w59, index (row)=1) -> (element=w49:dbl[])  [unwired: 1 in]
      n24 = Fract/Exp String To Number(string=w20) -> (number=w12:dbl[])  [unwired: 3 in, 1 out]
      n25 = Fract/Exp String To Number(string=w21) -> (number=w11:dbl[])  [unwired: 3 in, 1 out]
      n26 = Fract/Exp String To Number(string=w22) -> (number=w10:dbl[])  [unwired: 3 in, 1 out]
      n27 = Index Array(array=w59, index (row)=1) -> (element=w48:dbl[])  [unwired: 1 in]
      n28 = Fract/Exp String To Number(string=w28) -> (number=w27:dbl[])  [unwired: 3 in, 1 out]
      n29 = Fract/Exp String To Number(string=w26) -> (number=w25:dbl[])  [unwired: 3 in, 1 out]
      n30 = Fract/Exp String To Number(string=w24) -> (number=w23:dbl[])  [unwired: 3 in, 1 out]
      n31 = Index Array(array=w44, index (row)=0) -> (element=w38:dbl[])  [unwired: 1 in]
      n32 = Index Array(array=w44, index (row)=1) -> (element=w39:dbl[])  [unwired: 1 in]
      n33 = Bundle("all rows"=w34, "all rows"=w48) -> (w51:cluster{"all rows":dbl[], "all rows":dbl[]})  [unwired: 1 in]
      n34 = Bundle("all rows"=w34, "all rows"=w49) -> (w52:cluster{"all rows":dbl[], "all rows":dbl[]})  [unwired: 1 in]
      n35 = Bundle("all rows"=w36, "all rows"=w50) -> (w53:cluster{"all rows":dbl[], "all rows":dbl[]})  [unwired: 1 in]
      n36 = Bundle(w27, w23) -> (w65:cluster{dbl[], dbl[]})  [unwired: 1 in]
      n37 = Bundle(w27, w25) -> (w66:cluster{dbl[], dbl[]})  [unwired: 1 in]
      n38 = Bundle(w12, w10) -> (w67:cluster{dbl[], dbl[]})  [unwired: 1 in]
      n39 = Bundle(w12, w11) -> (w68:cluster{dbl[], dbl[]})  [unwired: 1 in]
      n40 = Build Array(w53, w52, w51) -> ()  [unwired: 1 out]
      n41 = expression code="x/1e9"(w34) -> (w33:dbl[])
      n42 = Build Array(w68, w67, w66, w65) -> ()  [unwired: 1 out]
      n43 = expression code="x/1e9"(w36) -> (w35:dbl[])
      n44 = call <vilib>:"Interpolate 1D.vi"("method"=w31, "xi"=w27, "X"=w33, "Y"=w49) -> ("yi"=w46:dbl[])  [unwired: 5 in, 2 out]
      n45 = call <vilib>:"Interpolate 1D.vi"("method"=w31, "xi"=w27, "X"=w33, "Y"=w48) -> ("yi"=w45:dbl[])  [unwired: 5 in, 2 out]
      n46 = call <vilib>:"Interpolate 1D.vi"("method"=w31, "xi"=w27, "X"=w35, "Y"=w50) -> ("yi"=w47:dbl[])  [unwired: 5 in, 2 out]
      n47 = call <vilib>:"Interpolate 1D.vi"("method"=2, "xi"=w27, "X"=w38, "Y"=w39) -> ("yi"=w37:dbl[])  [unwired: 5 in, 2 out]
      n48 = Build Array(w27, w25, w23, w11, w10, w47, w46, w45, w37) -> (w30:dbl[][])
      n49 = local write "配列"(w30) -> ()
    }
    frame #2 {
      n50 = local read "Calc_IFout"() -> (w74:T1)
      n51 = Unbundle By Name(w74) -> ("Th"=w76:dbl, "Tc"=w75:dbl)
      n52 = local read "配列"() -> (w81:dbl[][])
      n53 = Index Array(array=w81, index (row)=1) -> (element=w100:dbl[])  [unwired: 1 in]
      n54 = Index Array(array=w81, index (row)=3) -> (element=w94:dbl[])  [unwired: 1 in]
      n55 = Index Array(array=w81, index (row)=2) -> (element=w98:dbl[])  [unwired: 1 in]
      n56 = Index Array(array=w81, index (row)=4) -> (element=w92:dbl[])  [unwired: 1 in]
      n57 = Index Array(array=w81, index (row)=8) -> (element=w89:dbl[])  [unwired: 1 in]
      n58 = call "ダイナミックデータへ変換6"("Array"=w89) -> ("Dynamic Data Type"=w88:dynamicdata)  [unwired: 3 in]
      n59 = Transpose 2D Array(2D array=w81) -> (transposed array=w82:dbl[][])
      n60 = xnode "フォーミュラ5"("ENR"=w88, "Troom"=w76) -> ("結果"=w78:dynamicdata)  [unwired: 1 in, 1 out]
      n61 = call "___2ddata_to_multigraph.vi"("列"=i32[] [0, 1, 2, 3, 4, 5, 7, 8], "データ配列"=w82) -> ("XYグラフ"=→"XYグラフ 6":cluster{"データ配列":dbl[], "データ配列":dbl[]}[])  [unwired: 5 in]
      n62 = call "ダイナミックデータへ変換8"("Array"=w100) -> ("Dynamic Data Type"=w99:dynamicdata)  [unwired: 3 in]
      n63 = call "ダイナミックデータへ変換9"("Array"=w94) -> ("Dynamic Data Type"=w93:dynamicdata)  [unwired: 3 in]
      n64 = call "ダイナミックデータへ変換10"("Array"=w92) -> ("Dynamic Data Type"=w91:dynamicdata)  [unwired: 3 in]
      n65 = call "ダイナミックデータへ変換7"("Array"=w98) -> ("Dynamic Data Type"=w97:dynamicdata)  [unwired: 3 in]
      n66 = xnode "フォーミュラ4"("Ph"=w99, "Pc"=w97, "th"=w76, "tc"=w75) -> ("結果"=w87:dynamicdata)  [unwired: 1 in, 1 out]
      n67 = xnode "フォーミュラ6"("Ph"=w93, "Pc"=w91, "th"=w78, "tc"=w76) -> ("結果"=w85:dynamicdata)  [unwired: 1 in, 1 out]
      n68 = call "ダイナミックデータから変換4"("Dynamic Data Type"=w87) -> ("Array"=w86:dbl[])  [unwired: 3 in]
      n69 = call "ダイナミックデータから変換5"("Dynamic Data Type"=w85) -> ("Array"=w84:dbl[])  [unwired: 3 in]
      n70 = call "ダイナミックデータから変換6"("Dynamic Data Type"=w78) -> ("Array"=w77:dbl[])  [unwired: 3 in]
      n71 = Build Array (concatenate)(w81, w86, w84, w77) -> (w80:dbl[][])
      n72 = Transpose 2D Array(2D array=w80) -> (transposed array=w79:dbl[][])
      n73 = call "___2ddata_to_multigraph.vi"("列"=i32[] [0, 9, 10], "データ配列"=w79) -> ()  [unwired: 5 in, 1 out]
      n74 = local write "配列"(w80) -> ()
    }
    frame #3 {
      w527 = 0
      n75 = local read "配列"() -> (w528:dbl[][])
      n76 = Index Array(array=w528, index (row)=w527, index (col)=w527) -> (element=w525:dbl)
      n77 = Index Array(array=w528, index (row)=0, index (col)=1) -> (element=w526:dbl)
      n78 = Index Array(array=w528, index (row)=3) -> (element=w545:dbl[])  [unwired: 1 in]
      n79 = Index Array(array=w528, index (row)=1) -> (element=w533:dbl[])  [unwired: 1 in]
      n80 = Index Array(array=w528, index (row)=2) -> (element=w532:dbl[])  [unwired: 1 in]
      n81 = Index Array(array=w528, index (row)=5) -> (element=w544:dbl[])  [unwired: 1 in]
      n82 = Index Array(array=w528, index (row)=11) -> (element=w542:dbl[])  [unwired: 1 in]
      n83 = Index Array(array=w528, index (row)=7) -> (element=w543:dbl[])  [unwired: 1 in]
      n84 = Subtract(x=w526, y=w525) -> (x-y=w522:dbl)
      n85 = call "ダイナミックデータへ変換12"("Array"=w545) -> ("Dynamic Data Type"=w539:dynamicdata)  [unwired: 3 in]
      n86 = call "ダイナミックデータへ変換13"("Array"=w544) -> ("Dynamic Data Type"=w538:dynamicdata)  [unwired: 3 in]
      n87 = call "ダイナミックデータへ変換14"("Array"=w543) -> ("Dynamic Data Type"=w537:dynamicdata)  [unwired: 3 in]
      n88 = call "ダイナミックデータへ変換16"("Array"=w542) -> ("Dynamic Data Type"=w536:dynamicdata)  [unwired: 3 in]
      n89 = xnode "フォーミュラ"("Pnson"=w539, "kb"=1.38e-23, "Tnson"=w536, "bw"=w522, "Gamp"=w537, "Ginput"=w538) -> ("結果"=w534:dynamicdata)  [unwired: 1 in, 1 out]
      n90 = call "ダイナミックデータから変換"("Dynamic Data Type"=w534) -> ("Array"=w531:dbl[])  [unwired: 3 in]
      n91 = Add(x=w531, y=w533) -> (x+y=w530:dbl[])
      n92 = Add(x=w531, y=w532) -> (x+y=w529:dbl[])
      n93 = Build Array (concatenate)(w528, w530, w529) -> (w540:dbl[][])
      n94 = Transpose 2D Array(2D array=w540) -> (transposed array=w551:dbl[][])
      n95 = call "___2ddata_to_multigraph.vi"("列"=i32[] [0, 12, 13, 9], "データ配列"=w551) -> ("XYグラフ"=→"XYグラフ 4":cluster{"データ配列":dbl[], "データ配列":dbl[]}[])  [unwired: 5 in]
      n96 = local write "配列"(w540) -> ()
    }
    frame #4 {
      w720 = 0.0
      n97 = local read "Calc_IFout"() -> (w693:T1)
      n98 = Unbundle By Name(w693) -> ("Th"=w699:dbl, "Tc"=w698:dbl)
      n99 = local read "配列"() -> (w707:dbl[][])
      n100 = Index Array(array=w707, index (row)=12) -> (element=w709:dbl[])  [unwired: 1 in]
      n101 = Index Array(array=w707, index (row)=0) -> (element=w717:dbl[])  [unwired: 1 in]
      n102 = Index Array(array=w717, index=1) -> (element=w716:dbl)
      n103 = Index Array(array=w717, index=0) -> (element=w715:dbl)
      n104 = Index Array(array=w707, index (row)=13) -> (element=w708:dbl[])  [unwired: 1 in]
      n105 = Subtract(x=w716, y=w715) -> (x-y=w714:dbl)
      n106 = expression code="x*1e3"(w714) -> (w713:dbl)
      n107 = Array Size(array=w709) -> (size(s)=w722:i32)
      n108 = Divide(x=w713, y=1) -> (x/y=w705:dbl)
      n109 = for {
        N: w722 -> [_]
        tunnel: w717 -> [w750]
        tunnel: w708 -> [w744]
        shift-right: [w742] -> w712
        shift-left: w720 -> [w743]
        shift-right: [w740] -> w704
        shift-left: w720 -> [w741]
        tunnel: w709 -> [w739]
        tunnel: [w738] -> w697 mode=indexing
        i -> [w745]
        n110 = Index Array(array=w750, index=w745) -> (element=w749:dbl)
        n111 = In Range and Coerce(upper limit=12, x=w749, lower limit=4) -> (In Range?=w746:bool)  [unwired: 1 out]
        n112 = case shown="참" w746 {
          tunnel: w745 -> [_ w754]
          tunnel: w744 -> [_ w763]
          tunnel: w743 -> [w752 w760]
          tunnel: [w752 w759] -> w742
          tunnel: w741 -> [w751 w755]
          tunnel: [w751 w756] -> w740
          tunnel: w739 -> [_ w757]
          tunnel: [_ w753] -> w738
          frame False {
          }
          frame True {
            n113 = Index Array(array=w757, index=w754) -> (element=w753:dbl)
            n114 = Index Array(array=w763, index=w754) -> (element=w762:dbl)
            n115 = expression code="10**(x/10)"(w753) -> (w758:dbl)
            n116 = expression code="10**(x/10)"(w762) -> (w761:dbl)
            n117 = Add(x=w758, y=w755) -> (x+y=w756:dbl)
            n118 = Add(x=w761, y=w760) -> (x+y=w759:dbl)
          }
        }
      }
      n119 = Multiply(x=w712, y=w705) -> (x*y=w711:dbl)
      n120 = Multiply(x=w704, y=w705) -> (x*y=w706:dbl)
      n121 = expression code="log(x)*10"(w711) -> (w702:dbl)
      n122 = expression code="log(x)*10"(w706) -> (w703:dbl)
      n123 = local write "PrxCold(dBm)"(w702) -> ()
      n124 = local write "PrxHOT(dBm)"(w703) -> ()
      n125 = xnode "フォーミュラ2"("Ph"=w703, "Pc"=w702, "th"=w699, "tc"=w698) -> ("結果"=w701:dbl)  [unwired: 1 in, 1 out]
      n126 = local write "Trx(K)"(w701) -> ()
      n127 = Array Max & Min(array=w697) -> (max value=w696:dbl, min value=w695:dbl)  [unwired: 2 out]
      n128 = Subtract(x=w696, y=w695) -> (x-y=w694:dbl)
      n129 = local write "Inband PP"(w694) -> ()
    }
    frame #5 {
      n130 = local read "配列"() -> (w769:dbl[][])
      n131 = Index Array(array=w769, index (row)=12) -> (element=w772:dbl[])  [unwired: 1 in]
      n132 = Index Array(array=w769, index (row)=0) -> (element=w775:dbl[])  [unwired: 1 in]
      n133 = Index Array(array=w775, index=1) -> (element=w774:dbl)
      n134 = Index Array(array=w775, index=0) -> (element=w773:dbl)
      n135 = Subtract(x=w774, y=w773) -> (x-y=w771:dbl)
      n136 = Reciprocal(x=w771) -> (1/x=w770:dbl)
      n137 = Array Size(array=w772) -> (size(s)=w779:i32)
      n138 = for {
        N: w779 -> [_]
        tunnel: w775 -> [w789]
        tunnel: w772 -> [w783]
        tunnel: w770 -> [w782]
        tunnel: [w781] -> w768 mode=indexing
        i -> [w784]
        n139 = Index Array(array=w789, index=w784) -> (element=w788:dbl)
        n140 = In Range and Coerce(upper limit=11.0, x=w788, lower limit=5.0) -> (In Range?=w785:bool)  [unwired: 1 out]
        n141 = case shown="참" w785 {
          tunnel: w784 -> [_ w800]
          tunnel: w783 -> [_ w801]
          tunnel: w782 -> [_ w798]
          tunnel: [0.0 w793] -> w781
          frame False {
          }
          frame True {
            n142 = Subtract(x=w800, y=w798) -> (x-y=w799:dbl)
            n143 = Multiply(x=w798, y=2) -> (x*y=w792:dbl)
            n144 = Increment(x=w792) -> (x+1=w791:dbl)
            n145 = Array Subset(array=w801, index=w799, length=w791) -> (w796:dbl[])
            n146 = Array Max & Min(array=w796) -> (max value=w795:dbl, min value=w794:dbl)  [unwired: 2 out]
            n147 = Subtract(x=w795, y=w794) -> (x-y=w793:dbl)
          }
        }
      }
      n148 = Build Array (concatenate)(w769, w768) -> (w764:dbl[][])
      n149 = Transpose 2D Array(2D array=w764) -> (transposed array=w765:dbl[][])
      n150 = local write "配列"(w764) -> ()
      n151 = call "___2ddata_to_multigraph.vi"("列"=i32[] [0, 12, 14], "データ配列"=w765) -> ("XYグラフ"=→"XYグラフ 7":cluster{"データ配列":dbl[], "データ配列":dbl[]}[])  [unwired: 5 in]
    }
    frame #6 {
      n152 = local read "Calc_IFout"() -> (w803:T1)
      n153 = Unbundle By Name(w803) -> ("SAVE"=w805:bool, "Rx_output_data"=w804:path)
      n154 = case shown="참" w805 {
        tunnel: w804 -> [_ w806]
        frame False {
        }
        frame True {
          n155 = stacked-sequence {
            tunnel: w806 -> [w807 w825 w894]
            frame #0 {
              n156 = local read "配列"() -> (w812:dbl[][])
              n157 = Strip Path(path=w807) -> (stripped path=w810:path, name=w808:string)
              n158 = Concatenate Strings("A_", w808) -> (w811:string)
              n159 = call "___save_2d_data_with_header.vi"("ヘッダー"="IF,Ph,Pc,Pnson,Pnsoff,Ginput,dummy,Gnsamp,NSenr,Trx_cart,Trx_ifbox,Tnson,PoutH,PoutC,PP", "配列"=w812, "形式"="%.3f", "file_name"=w811, "パス"=w810) -> ()  [unwired: 6 in, 1 out]
            }
            frame #1 {
              n160 = local read "配列"() -> (w823:dbl[][])
              n161 = Strip Path(path=w825) -> (stripped path=w820:path, name=w826:string)
              n162 = Index Array(array=w823, index (row)=0) -> (element=w817:dbl[])  [unwired: 1 in]
              n163 = Array Size(array=w817) -> (size(s)=w822:i32)
              n164 = Concatenate Strings("PV_", w826) -> (w821:string)
              n165 = Build Path(base path=w820, name or relative path=w821) -> (appended path=w819:path)
              n166 = Open/Create/Replace File(file path (use dialog)=w819, operation (0:open)=4) -> (refnum out=w818:refnum<file>)  [unwired: 4 in, 2 out]
              n167 = stacked-sequence {
                tunnel: w822 -> [_ w845]
                tunnel: w818 -> [_ w844]
                tunnel: w817 -> [_ w843]
                tunnel: [_ w842] -> w815
                frame #0 {
                  w836 = 0
                  n168 = local read "文字列配列"() -> (w841:string[][])
                  n169 = local read "Inband PP"() -> (w834:dbl)
                  n170 = Index Array(array=w841, index (row)=0, index (col)=w836) -> (element=w832:string)
                  n171 = Index Array(array=w841, index (row)=1, index (col)=w836) -> (element=w831:string)
                  n172 = Index Array(array=w841, index (row)=4, index (col)=w836) -> (element=w830:string)
                  n173 = Index Array(array=w841, index (row)=5, index (col)=w836) -> (element=w829:string)
                  n174 = local read "Trx(K)"() -> (w828:dbl)
                  n175 = Format Into String(format string="PV_tot,%s,%s,%s,%s,0.00,8.00,%.2f \nNT_tot,%s,%s,0.00,8.00,%s,%s,%.2f ", w832, w831, w830, w829, w834, w832, w831, w830, w829, w828) -> (resulting string=w833:string)  [unwired: 2 in, 1 out]
                  n176 = local write "出力文字列"(w833) -> ()
                }
                frame #1 {
                  n177 = for {
                    N: w845 -> [_]
                    tunnel: w844 -> [w867]
                    tunnel: w843 -> [w862]
                    tunnel: [w853] -> w842
                    i -> [w846]
                    n178 = local read "文字列配列"() -> (w860:string[][])
                    n179 = local read "配列"() -> (w866:dbl[][])
                    n180 = Index Array(array=w860, index (row)=0, index (col)=w846) -> (element=w859:string)
                    n181 = Index Array(array=w860, index (row)=1, index (col)=w846) -> (element=w858:string)
                    n182 = Index Array(array=w860, index (row)=4, index (col)=w846) -> (element=w857:string)
                    n183 = Index Array(array=w866, index (row)=14, index (col)=w846) -> (element=w854:dbl)
                    n184 = Index Array(array=w860, index (row)=5, index (col)=w846) -> (element=w856:string)
                    n185 = Index Array(array=w860, index (row)=2, index (col)=w846) -> (element=w855:string)
                    n186 = Index Array(array=w862, index=w846) -> (element=w865:dbl)
                    n187 = In Range and Coerce(upper limit=11.0, x=w865, lower limit=5.0) -> (In Range?=w861:bool)  [unwired: 1 out]
                    n188 = case shown="참" w861 {
                      tunnel: w867 -> [w868 w877]
                      tunnel: w859 -> [_ w875]
                      tunnel: w858 -> [_ w874]
                      tunnel: w857 -> [_ w873]
                      tunnel: w856 -> [_ w872]
                      tunnel: w855 -> [_ w871]
                      tunnel: w854 -> [_ w870]
                      tunnel: [w868 w869] -> w853
                      frame False {
                      }
                      frame True {
                        n189 = Format Into String(format string="%s ,%s ,%s ,%s , %s, 2.0,%.2f \\n", initial string=w877, w875, w874, w873, w872, w871, w870) -> (resulting string=w869:refnum<file>)  [unwired: 1 in, 1 out]
                      }
                    }
                  }
                }
              }
              n190 = Close File(refnum=w815) -> ()  [unwired: 1 in, 2 out]
            }
            frame #2 {
              w884 = 0
              n191 = local read "配列"() -> (w879:dbl[][])
              n192 = Strip Path(path=w894) -> (stripped path=w890:path, name=w895:string)
              n193 = Index Array(array=w879, index (row)=0) -> (element=w887:dbl[])  [unwired: 1 in]
              n194 = Array Size(array=w887) -> (size(s)=w892:i32)
              n195 = Concatenate Strings("IFS_", w895) -> (w891:string)
              n196 = Build Path(base path=w890, name or relative path=w891) -> (appended path=w889:path)
              n197 = Open/Create/Replace File(file path (use dialog)=w889, operation (0:open)=4) -> (refnum out=w888:refnum<file>)  [unwired: 4 in, 2 out]
              n198 = Index Array(array=w879, index (row)=w884, index (col)=w884) -> (element=w882:dbl)
              n199 = Index Array(array=w879, index (row)=0, index (col)=1) -> (element=w883:dbl)
              n200 = Subtract(x=w883, y=w882) -> (x-y=w878:dbl)
              n201 = for {
                N: w892 -> [_]
                tunnel: w888 -> [w915]
                tunnel: w887 -> [_]
                tunnel: [w908] -> w886
                tunnel: w878 -> [w900]
                i -> [w901]
                n202 = local read "文字列配列"() -> (w914:string[][])
                n203 = local read "配列"() -> (w897:dbl[][])
                n204 = Index Array(array=w914, index (row)=0, index (col)=w901) -> (element=w913:string)
                n205 = Index Array(array=w914, index (row)=1, index (col)=w901) -> (element=w912:string)
                n206 = Index Array(array=w914, index (row)=4, index (col)=w901) -> (element=w911:string)
                n207 = Index Array(array=w897, index (row)=12, index (col)=w901) -> (element=w898:dbl)
                n208 = Index Array(array=w914, index (row)=5, index (col)=w901) -> (element=w910:string)
                n209 = Index Array(array=w914, index (row)=2, index (col)=w901) -> (element=w909:string)
                n210 = Format Into String(format string="%s,%s,%s,%s,%s,%.2f,%.2f \\n", initial string=w915, w913, w912, w911, w910, w909, w900, w898) -> (resulting string=w908:refnum<file>)  [unwired: 1 in, 1 out]
              }
              n211 = Close File(refnum=w886) -> ()  [unwired: 1 in, 2 out]
            }
          }
        }
      }
      n212 = local read "Calc_IFout"() -> (w802:T1)
      n213 = local write "Calc_IFout 2"(w802) -> ()
    }
  }
